vi "单参数加标流程.vi"(10 "流程类型":T4, 11 "Slave ID":T6=enum."氨氮") -> ()   [LabVIEW 2016, in "质控单元V4.lvlib"]
panel:
  in  "平行样测试数据":T1={"时间"=timestamp(0 s since 1904-01-01), "参数"="", "数据类型"="N", "第一次水样浓度值"=0.0, "第二次水样测试时间"=timestamp(0 s since 1904-01-01), "第二次水样浓度值"=0.0}
  in  "集成干预测试数据":T2={"时间"=timestamp(0 s since 1904-01-01), "参数"="", "数据类型"="N", "集成干预测试浓度值"=0.0, "集成干预前测试时间"=timestamp(0 s since 1904-01-01), "集成干预前测试浓度值"=0.0}
  out "平行样启动时间":timestamp
  out "加标模块润洗流程控制":T3=enum."启动水样润洗流程"
  in  "获取加标回收测试数据计数":u16
  in  "获取水样测试数据计数":u16
  in  "写入加标体积重试次数":u16
  in  "加标模块加标润洗启动计数":u16
  out "加标回收启动时间":timestamp
  out "水样测试启动时间":timestamp
  out "Next State":string
  in  "仪器加标回收启动计数":u16
  in  "仪器水样测试启动计数":u16
  in  "加标模块排液启动计数":u16
  in  "加标模块加标启动计数":u16
  in  "加标模块进样启动计数":u16
  in  "加标模块水样润洗启动计数":u16
  in  "采配水启动次数计数":u16
  in  "加标回收测试时间":timestamp
  in  "水样测试时间":timestamp
  in  "质控数据":T5
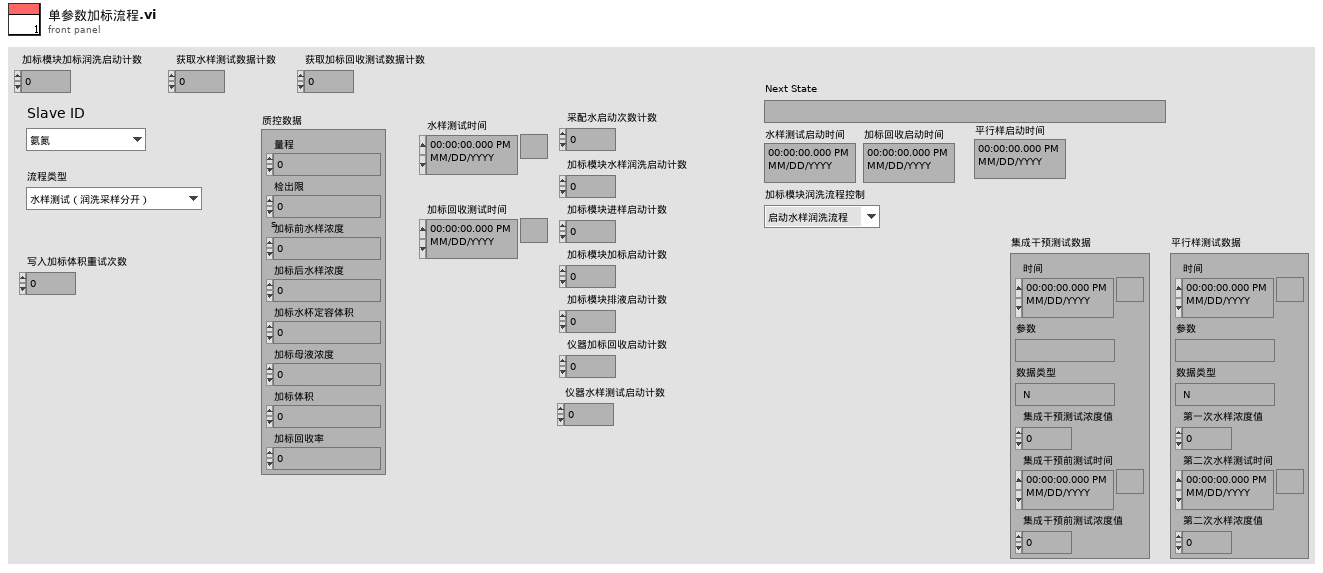
[diagram p1: front panel]
types:
  T1 = typedef "平行样测试数据字段定义.ctl" = cluster{"时间":timestamp, "参数":string, "数据类型":string, "第一次水样浓度值":dbl, "第二次水样测试时间":timestamp, "第二次水样浓度值":dbl}
  T2 = typedef "集成干预字段定义.ctl" = cluster{"时间":timestamp, "参数":string, "数据类型":string, "集成干预测试浓度值":dbl, "集成干预前测试时间":timestamp, "集成干预前测试浓度值":dbl}
  T3 = typedef "质控单元V4.lvlib/质控流程控制.ctl" = enum16{"待机", "启动进样流程", "启动加标流程", "启动排液流程", "启动水样润洗流程", "启动加标润洗流程", "停止流程"}
  T4 = typedef "质控单元V4.lvlib/测试子流程.ctl" = enum16{"水样测试（润洗采样分开）", "水样测试（润洗采样合并）", "水样测试（不启动采配水）", "加标回收（润洗采样分开）", "加标回收（润洗采样合并）", "加标回收（不启动采配水）", "集成干预测试", "平行样测试", "平行样测试（不启动采配水）", "水样测试（不含采样杯）", "平行样测试（不含采样杯）", "集成干预测试（不含采样杯）"}
  T5 = cluster{"量程":dbl, "检出限":dbl, "加标前水样浓度":dbl, "加标后水样浓度":dbl, "加标水杯定容体积":dbl, "加标母液浓度":dbl, "加标体积":dbl, "加标回收率":dbl}
  T6 = typedef "质控单元V4.lvlib/质控slave id.ctl" = enum16{"null", "氨氮", "总磷", "总氮", "CODMn", "CODCr"}
  T7 = cluster{"氨氮":bool, "总磷":bool, "总氮":bool, "CODMn":bool, "CODCr":bool}
  T8 = cluster{"时间":timestamp, "参数":string, "数据类型":string, "加标回收率":sgl, "加标前水样测试时间":timestamp, "加标前水样浓度值":sgl, "加标后水样浓度值":sgl, "加标母液浓度值":sgl, "加标体积":sgl, "加标水杯定容体积":sgl}
  T9 = enum16{"待机", "水样测试（全流程）", "停止", "加标回收", "水样测试（简易流程）"}
  T10 = enum16{"待机", "润洗", "采样", "沉淀", "配水", "反冲洗", "储水", "结束"}
  T11 = typedef "质控单元V4.lvlib/采配水通用流程.ctl" = enum16{"待机", "润洗", "采样", "沉淀", "配水", "反冲洗", "结束"}
  T12 = typedef "质控单元V4.lvlib/质控组合命令区.ctl" = enum16{"停止", "进水样", "排废液", "进空气（搅拌）", "定量（反转定量）"}
  T13 = enum16{"待机", "润洗", "进样", "定量", "加标", "等待取样", "排液", "异常停机"}
  T14 = enum16{"空闲", "水样测试", "标样核查", "零点核查", "跨度核查", "空白测试", "平行样测试", "加标回收", "空白校准", "标样校准", "初始化（清洗）"}
  T15 = cluster{"水样数据时间":timestamp, "水样实测值":sgl, "水样数据标识":string}
  T16 = cluster{"时间":timestamp, "参数":string, "数据类型":string, "第一次水样浓度值":dbl, "第二次水样测试时间":timestamp, "第二次水样浓度值":dbl}
  T17 = typedef "数据库类型.ctl" = enum16{"Access", "SQLite"}
  T18 = cluster{"加标回收数据时间":timestamp, "加标回收实测值":sgl, "加标回收数据标识":string}
  T19 = typedef "质控单元V4.lvlib/质控仪器状态.ctl" = cluster{"运行状态":enum16{"待机", "润洗", "进样", "定量", "加标", "等待取样", "排液", "异常停机"}, "液位状态":enum16{"无感应", "有感应"}, "告警状态":enum16{"无告警", "液位故障告警", "注射泵异常"}, "当前步骤数":u16, "当前步骤剩余时间":u16, "当前步骤具体操作":enum16{"加标", "进样", "排液", "搅拌", "定量"}, "当前流程":enum16{"待机", "进样流程", "加标流程", "排液流程", "水样润洗流程", "加标润洗流程"}}
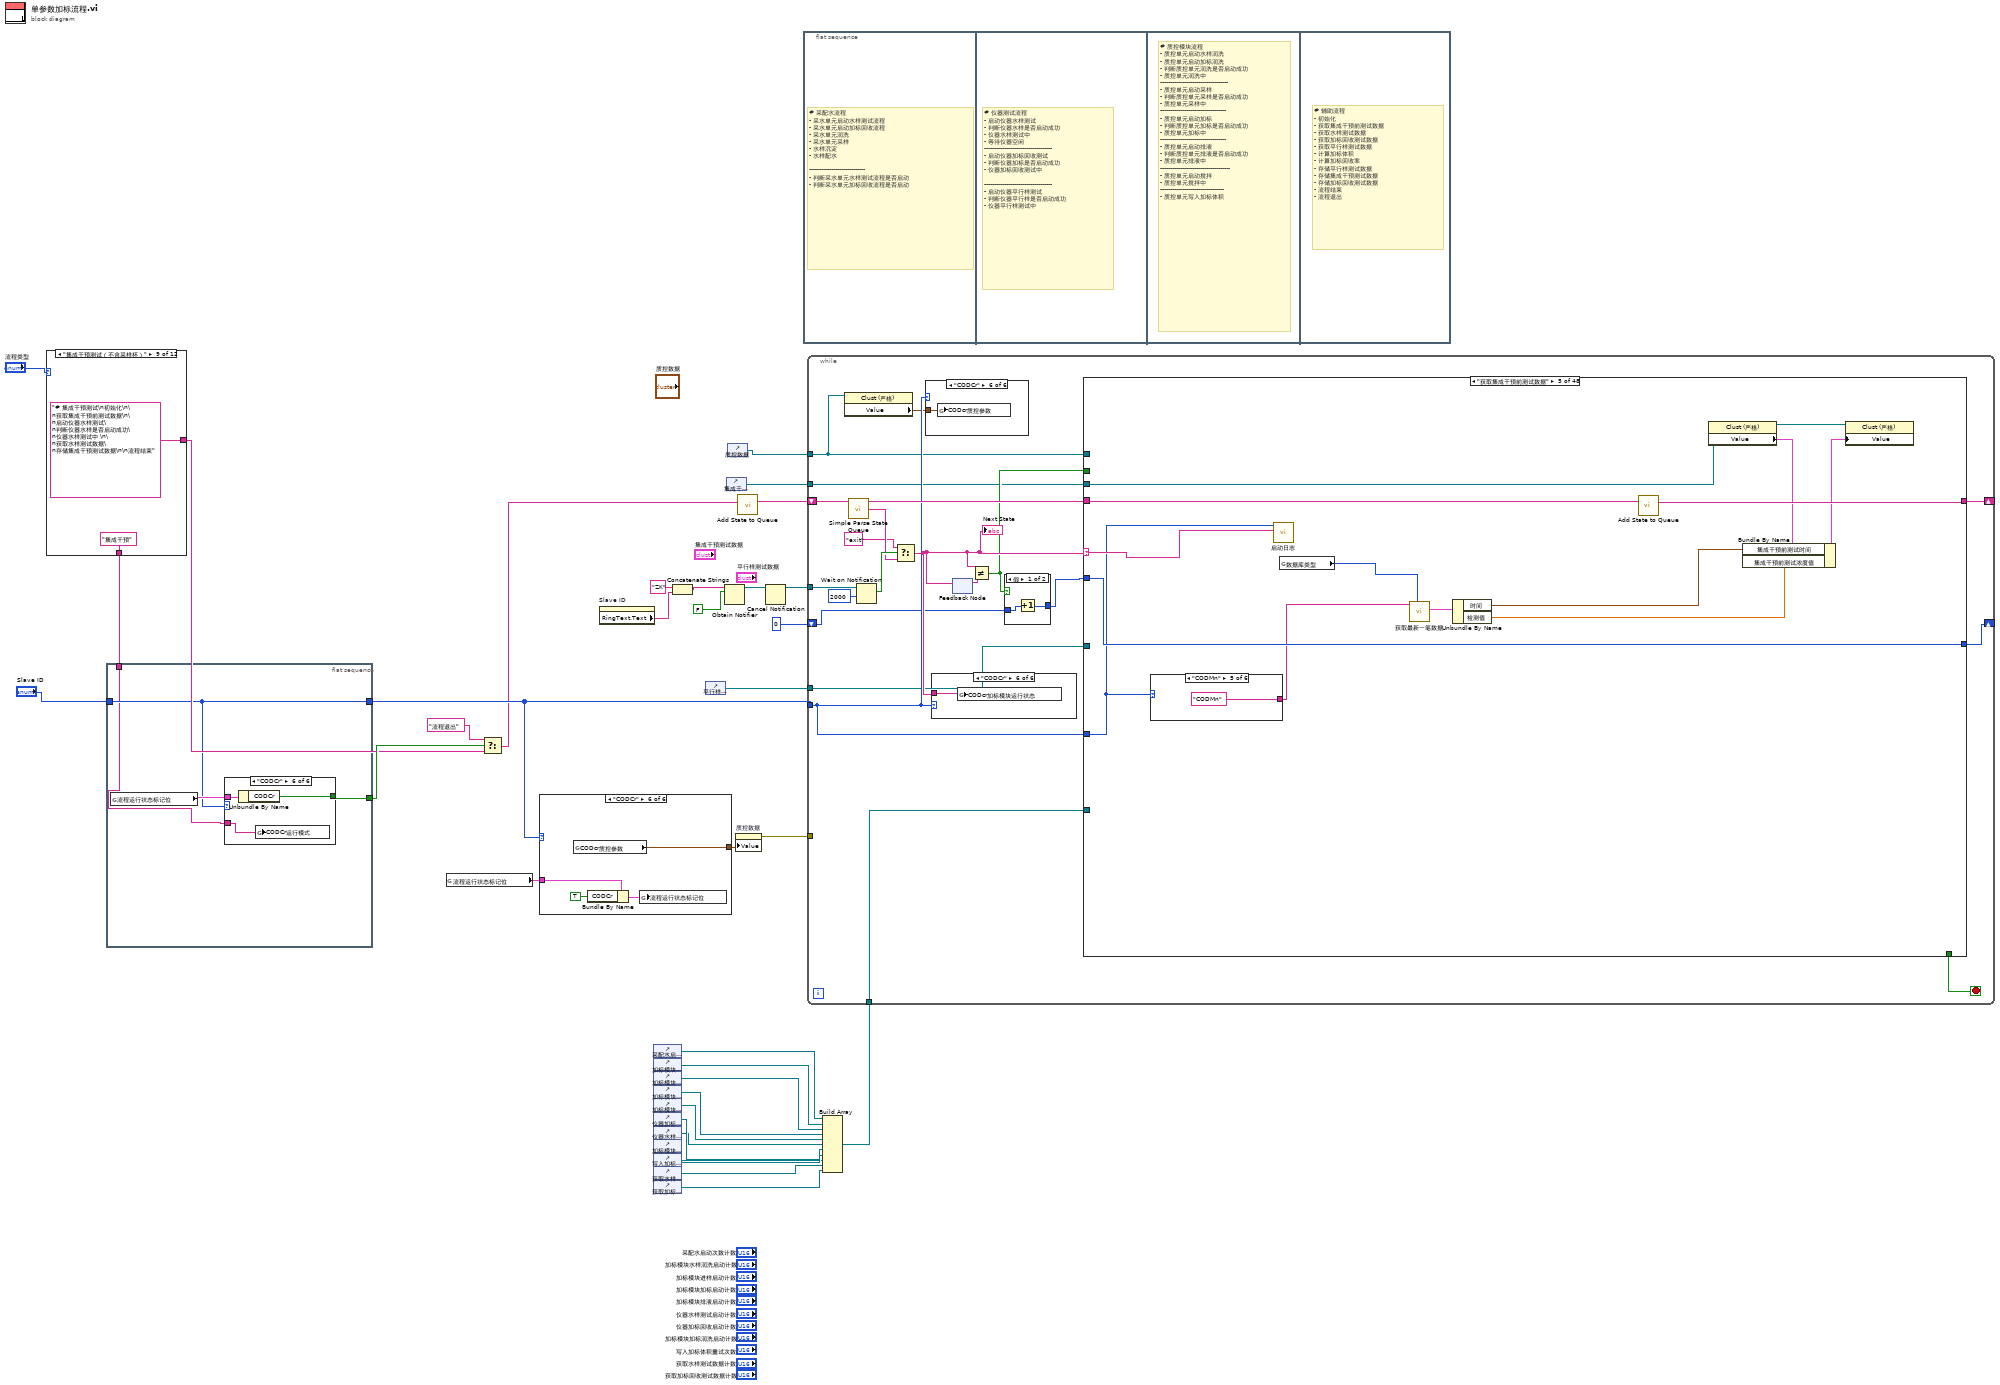
[diagram p0: block diagram]
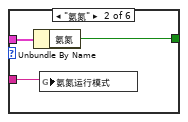
[diagram p3: hidden frame]
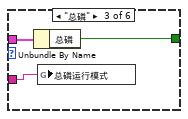
[diagram p4: hidden frame]
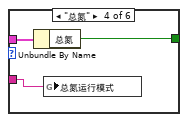
[diagram p5: hidden frame]
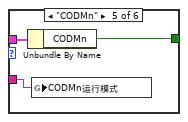
[diagram p6: hidden frame]
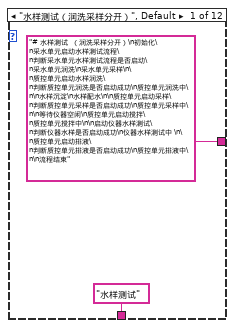
[diagram p7: hidden frame]
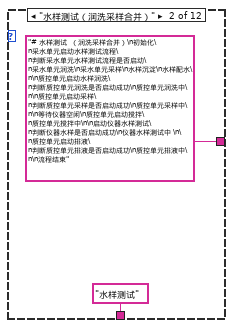
[diagram p8: hidden frame]
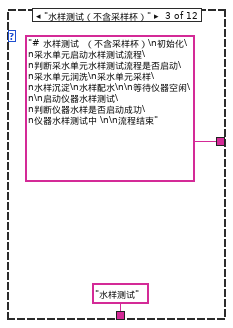
[diagram p9: hidden frame]
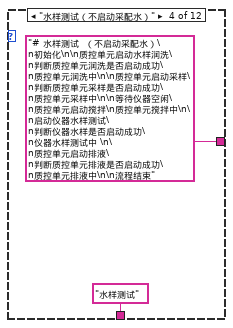
[diagram p10: hidden frame]
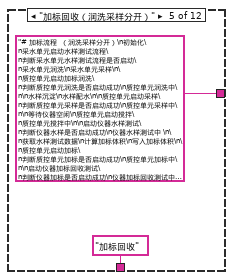
[diagram p11: hidden frame]
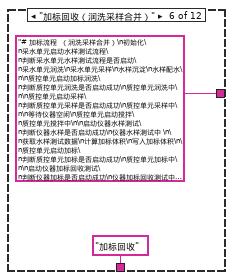
[diagram p12: hidden frame]
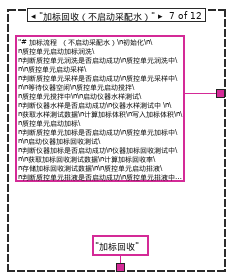
[diagram p13: hidden frame]
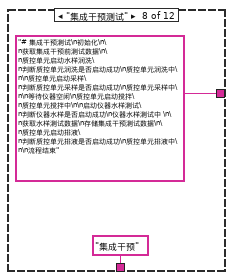
[diagram p14: hidden frame]
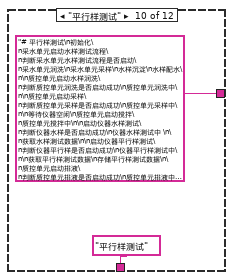
[diagram p15: hidden frame]
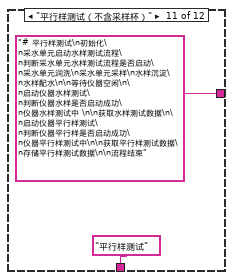
[diagram p16: hidden frame]
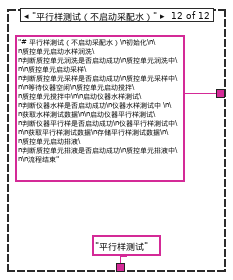
[diagram p17: hidden frame]
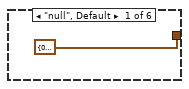
[diagram p18: hidden frame]
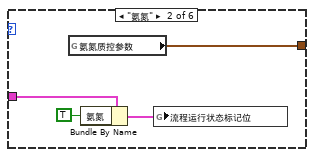
[diagram p19: hidden frame]
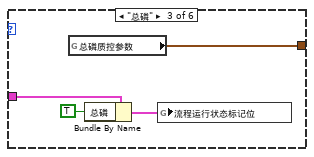
[diagram p20: hidden frame]
diagram:
  n1 = case shown="\"集成干预测试（不含采样杯）\"" "流程类型" {
    tunnel: ["# 水样测试  （润洗采样分开）\n初始化\n采水单元启动水样测试流程\n判断采水单元水样测试流程是否启动\n采水单元润洗\n采水单元采样\n\n质控单元启动水样润洗\n判断质控单元润洗是否启动成功\n质控单元润洗中\n\n水样沉淀\n水样配水\n\n质控单元启动采样\n判断质控单元采样是否启动成功\n质控单元采样中\n\n等待仪器空闲\n质控单元启动搅拌\n质控单元搅拌中\n\n启动仪器水样测试\n判断仪器水样是否启动成功\n仪器水样测试中 \n\n质控单元启动排液\n判断质控单元排液是否启动成功\n质控单元排液中\n\n流程结束" ("State(s) In (\"\")") "# 水样测试  （润洗采样合并）\n初始化\n采水单元启动水样测试流程\n判断采水单元水样测试流程是否启动\n采水单元润洗\n采水单元采样\n水样沉淀\n水样配水\n\n质控单元启动水样润洗\n判断质控单元润洗是否启动成功\n质控单元润洗中\n\n质控单元启动采样\n判断质控单元采样是否启动成功\n质控单元采样中\n\n等待仪器空闲\n质控单元启动搅拌\n质控单元搅拌中\n\n启动仪器水样测试\n判断仪器水样是否启动成功\n仪器水样测试中 \n\n质控单元启动排液\n判断质控单元排液是否启动成功\n质控单元排液中\n\n流程结束" ("State(s) In (\"\")") "# 水样测试  （不含采样杯）\n初始化\n采水单元启动水样测试流程\n判断采水单元水样测试流程是否启动\n采水单元润洗\n采水单元采样\n水样沉淀\n水样配水\n\n等待仪器空闲\n\n启动仪器水样测试\n判断仪器水样是否启动成功\n仪器水样测试中 \n\n流程结束" ("State(s) In (\"\")") "# 水样测试  （不启动采配水）\n初始化\n\n质控单元启动水样润洗\n判断质控单元润洗是否启动成功\n质控单元润洗中\n\n质控单元启动采样\n判断质控单元采样是否启动成功\n质控单元采样中\n\n等待仪器空闲\n质控单元启动搅拌\n质控单元搅拌中\n\n启动仪器水样测试\n判断仪器水样是否启动成功\n仪器水样测试中 \n\n质控单元启动排液\n判断质控单元排液是否启动成功\n质控单元排液中\n\n流程结束" ("State(s) In (\"\")") "# 加标流程  （润洗采样分开）\n初始化\n采水单元启动水样测试流程\n判断采水单元水样测试流程是否启动\n采水单元润洗\n采水单元采样\n\n质控单元启动加标润洗\n判断质控单元润洗是否启动成功\n质控单元润洗中\n\n水样沉淀\n水样配水\n\n质控单元启动采样\n判断质控单元采样是否启动成功\n质控单元采样中\n\n等待仪器空闲\n质控单元启动搅拌\n质控单元搅拌中\n\n启动仪器水样测试\n判断仪器水样是否启动成功\n仪器水样测试中 \n\n获取水样测试数据\n计算加标体积\n写入加标体积\n\n质控单元启动加标\n判断质控单元加标是否启动成功\n质控单元加标中\n\n启动仪器加标回收测试\n判断仪器加标是否启动成功\n仪器加标回收测试中\n\n获取加标回收测试数据\n计算加标回收率\n存储加标回收测试数据\n\n质控单元启动排液\n判断质控单元排液是否启动成功\n质控单元排液中\n\n流程结束" ("State(s) In (\"\")") "# 加标流程  （润洗采样合并）\n初始化\n采水单元启动水样测试流程\n判断采水单元水样测试流程是否启动\n采水单元润洗\n采水单元采样\n水样沉淀\n水样配水\n\n质控单元启动加标润洗\n判断质控单元润洗是否启动成功\n质控单元润洗中\n\n质控单元启动采样\n判断质控单元采样是否启动成功\n质控单元采样中\n\n等待仪器空闲\n质控单元启动搅拌\n质控单元搅拌中\n\n启动仪器水样测试\n判断仪器水样是否启动成功\n仪器水样测试中 \n\n获取水样测试数据\n计算加标体积\n写入加标体积\n\n质控单元启动加标\n判断质控单元加标是否启动成功\n质控单元加标中\n\n启动仪器加标回收测试\n判断仪器加标是否启动成功\n仪器加标回收测试中\n\n获取加标回收测试数据\n计算加标回收率\n存储加标回收测试数据\n\n质控单元启动排液\n判断质控单元排液是否启动成功\n质控单元排液中\n\n流程结束" ("State(s) In (\"\")") "# 加标流程  （不启动采配水）\n初始化\n\n质控单元启动加标润洗\n判断质控单元润洗是否启动成功\n质控单元润洗中\n\n质控单元启动采样\n判断质控单元采样是否启动成功\n质控单元采样中\n\n等待仪器空闲\n质控单元启动搅拌\n质控单元搅拌中\n\n启动仪器水样测试\n判断仪器水样是否启动成功\n仪器水样测试中 \n\n获取水样测试数据\n计算加标体积\n写入加标体积\n\n质控单元启动加标\n判断质控单元加标是否启动成功\n质控单元加标中\n\n启动仪器加标回收测试\n判断仪器加标是否启动成功\n仪器加标回收测试中\n\n获取加标回收测试数据\n计算加标回收率\n存储加标回收测试数据\n\n质控单元启动排液\n判断质控单元排液是否启动成功\n质控单元排液中\n\n流程结束" ("State(s) In (\"\")") "# 集成干预测试\n初始化\n\n获取集成干预前测试数据\n\n质控单元启动水样润洗\n判断质控单元润洗是否启动成功\n质控单元润洗中\n\n质控单元启动采样\n判断质控单元采样是否启动成功\n质控单元采样中\n\n等待仪器空闲\n质控单元启动搅拌\n质控单元搅拌中\n\n启动仪器水样测试\n判断仪器水样是否启动成功\n仪器水样测试中 \n\n获取水样测试数据\n存储集成干预测试数据\n\n质控单元启动排液\n判断质控单元排液是否启动成功\n质控单元排液中\n\n流程结束" ("State(s) In (\"\")") "# 集成干预测试\n初始化\n\n获取集成干预前测试数据\n\n启动仪器水样测试\n判断仪器水样是否启动成功\n仪器水样测试中 \n\n获取水样测试数据\n存储集成干预测试数据\n\n流程结束" ("State(s) In (\"\")") "# 平行样测试\n初始化\n采水单元启动水样测试流程\n判断采水单元水样测试流程是否启动\n采水单元润洗\n采水单元采样\n水样沉淀\n水样配水\n\n质控单元启动水样润洗\n判断质控单元润洗是否启动成功\n质控单元润洗中\n\n质控单元启动采样\n判断质控单元采样是否启动成功\n质控单元采样中\n\n等待仪器空闲\n质控单元启动搅拌\n质控单元搅拌中\n\n启动仪器水样测试\n判断仪器水样是否启动成功\n仪器水样测试中 \n\n获取水样测试数据\n\n启动仪器平行样测试\n判断仪器平行样是否启动成功\n仪器平行样测试中\n\n获取平行样测试数据\n存储平行样测试数据\n\n质控单元启动排液\n判断质控单元排液是否启动成功\n质控单元排液中\n\n流程结束" ("State(s) In (\"\")") "# 平行样测试\n初始化\n采水单元启动水样测试流程\n判断采水单元水样测试流程是否启动\n采水单元润洗\n采水单元采样\n水样沉淀\n水样配水\n\n等待仪器空闲\n\n启动仪器水样测试\n判断仪器水样是否启动成功\n仪器水样测试中 \n\n获取水样测试数据\n\n启动仪器平行样测试\n判断仪器平行样是否启动成功\n仪器平行样测试中\n\n获取平行样测试数据\n存储平行样测试数据\n\n流程结束" ("State(s) In (\"\")") "# 平行样测试（不启动采配水）\n初始化\n\n质控单元启动水样润洗\n判断质控单元润洗是否启动成功\n质控单元润洗中\n\n质控单元启动采样\n判断质控单元采样是否启动成功\n质控单元采样中\n\n等待仪器空闲\n质控单元启动搅拌\n质控单元搅拌中\n\n启动仪器水样测试\n判断仪器水样是否启动成功\n仪器水样测试中 \n\n获取水样测试数据\n\n启动仪器平行样测试\n判断仪器平行样是否启动成功\n仪器平行样测试中\n\n获取平行样测试数据\n存储平行样测试数据\n\n质控单元启动排液\n判断质控单元排液是否启动成功\n质控单元排液中\n\n流程结束" ("State(s) In (\"\")")] -> w12
    tunnel: ["水样测试" "水样测试" "水样测试" "水样测试" "加标回收" "加标回收" "加标回收" "集成干预" "集成干预" "平行样测试" "平行样测试" "平行样测试"] -> w6
    frame "水样测试（润洗采样分开）", Default {
    }
    frame "水样测试（润洗采样合并）" {
    }
    frame "水样测试（不含采样杯）" {
    }
    frame "水样测试（不启动采配水）" {
    }
    frame "加标回收（润洗采样分开）" {
    }
    frame "加标回收（润洗采样合并）" {
    }
    frame "加标回收（不启动采配水）" {
    }
    frame "集成干预测试" {
    }
    frame "集成干预测试（不含采样杯）" {
    }
    frame "平行样测试" {
    }
    frame "平行样测试（不含采样杯）" {
    }
    frame "平行样测试（不启动采配水）" {
    }
  }
  n2 = flat-sequence {
    tunnel: [w60] -> w15
    tunnel: [w61] -> w14
    tunnel: "Slave ID" -> [w60]
    tunnel: w6 -> [w59]
    frame #0 {
      n3 = global read "ZK非断电保存全局变量.vi" "流程运行状态标记位"() -> (w62:T7)
      n4 = case shown="\"CODCr\"" w60 {
        tunnel: w62 -> [_ w65 w68 w71 w74 w77]
        tunnel: [_ w64 w67 w70 w73 w76] -> w61
        tunnel: w59 -> [_ w63 w66 w69 w72 w75]
        frame "null", Default {
        }
        frame "氨氮" {
          n5 = Unbundle By Name(w65) -> ("氨氮"=w64:bool)
          n6 = global write "ZK非断电保存全局变量.vi" "氨氮运行模式"(w63) -> ()
        }
        frame "总磷" {
          n7 = Unbundle By Name(w68) -> ("总磷"=w67:bool)
          n8 = global write "ZK非断电保存全局变量.vi" "总磷运行模式"(w66) -> ()
        }
        frame "总氮" {
          n9 = Unbundle By Name(w71) -> ("总氮"=w70:bool)
          n10 = global write "ZK非断电保存全局变量.vi" "总氮运行模式"(w69) -> ()
        }
        frame "CODMn" {
          n11 = Unbundle By Name(w74) -> ("CODMn"=w73:bool)
          n12 = global write "ZK非断电保存全局变量.vi" "CODMn运行模式"(w72) -> ()
        }
        frame "CODCr" {
          n13 = Unbundle By Name(w77) -> ("CODCr"=w76:bool)
          n14 = global write "ZK非断电保存全局变量.vi" "CODCr运行模式"(w75) -> ()
        }
      }
    }
  }
  n15 = global read "ZK非断电保存全局变量.vi" "流程运行状态标记位"() -> (w17:T7)
  n16 = Select(t="流程退出", s=w14, f=w12) -> (s? t:f=w11:string)
  n17 = case shown="\"CODCr\"" w15 {
    tunnel: [T5 {"量程"=0.0, "检出限"=0.0, "加标前水样浓度"=0.0, "加标后水样浓度"=0.0, "加标水杯定容体积"=0.0, "加标母液浓度"=0.0, "加标体积"=0.0, "加标回收率"=0.0} ("CODcr质控参数") w82 w86 w90 w94 w98] -> w26
    tunnel: w17 -> [_ w81 w83 w87 w91 w95]
    frame "null", Default {
    }
    frame "氨氮" {
      n18 = global read "ZK断电保存全局变量.vi" "氨氮质控参数"() -> (w82:T5)
      n19 = Bundle By Name(cluster=w81, "氨氮"=TRUE) -> (w80:T7)
      n20 = global write "ZK非断电保存全局变量.vi" "流程运行状态标记位"(w80) -> ()
    }
    frame "总磷" {
      n21 = global read "ZK断电保存全局变量.vi" "总磷质控参数"() -> (w86:T5)
      n22 = Bundle By Name(cluster=w83, "总磷"=TRUE ("氨氮")) -> (w85:T7)
      n23 = global write "ZK非断电保存全局变量.vi" "流程运行状态标记位"(w85) -> ()
    }
    frame "总氮" {
      n24 = global read "ZK断电保存全局变量.vi" "总氮质控参数"() -> (w90:T5)
      n25 = Bundle By Name(cluster=w87, "总氮"=TRUE ("氨氮")) -> (w89:T7)
      n26 = global write "ZK非断电保存全局变量.vi" "流程运行状态标记位"(w89) -> ()
    }
    frame "CODMn" {
      n27 = global read "ZK断电保存全局变量.vi" "CODMn质控参数"() -> (w94:T5)
      n28 = Bundle By Name(cluster=w91, "CODMn"=TRUE ("氨氮")) -> (w93:T7)
      n29 = global write "ZK非断电保存全局变量.vi" "流程运行状态标记位"(w93) -> ()
    }
    frame "CODCr" {
      n30 = global read "ZK断电保存全局变量.vi" "CODcr质控参数"() -> (w98:T5)
      n31 = Bundle By Name(cluster=w95, "CODCr"=TRUE ("氨氮")) -> (w97:T7)
      n32 = global write "ZK非断电保存全局变量.vi" "流程运行状态标记位"(w97) -> ()
    }
  }
  n33 = property on="Slave ID" class="Enum (严格)"() -> ("RingText.Text"=w34:string)  [unwired: 2 in, 2 out]
  n34 = control-ref of="采配水启动次数计数"() -> (w24:refnum<vi>)
  n35 = control-ref of="加标模块水样润洗启动计数"() -> (w23:refnum<vi>)
  n36 = control-ref of="加标模块进样启动计数"() -> (w22:refnum<vi>)
  n37 = control-ref of="加标模块加标启动计数"() -> (w21:refnum<vi>)
  n38 = control-ref of="加标模块排液启动计数"() -> (w20:refnum<vi>)
  n39 = control-ref of="仪器加标回收启动计数"() -> (w5:refnum<vi>)
  n40 = control-ref of="仪器水样测试启动计数"() -> (w4:refnum<vi>)
  n41 = control-ref of="加标模块加标润洗启动计数"() -> (w16:refnum<vi>)
  n42 = control-ref of="写入加标体积重试次数"() -> (w10:refnum<vi>)
  n43 = control-ref of="获取水样测试数据计数"() -> (w9:refnum<vi>)
  n44 = control-ref of="获取加标回收测试数据计数"() -> (w8:refnum<vi>)
  n45 = Concatenate Strings("ZK" ("字符串"), w34) -> (w32:string)
  n46 = control-ref of="平行样测试数据"() -> (w1:refnum<vi>)
  n47 = Obtain Notifier(name (unnamed)=w32, notification data type=FALSE) -> (notifier out=w30:refnum<notifier>)  [unwired: 2 in, 2 out]
  n48 = control-ref of="集成干预测试数据"() -> (w2:refnum<vi>)
  n49 = control-ref of="质控数据"() -> (w25:refnum<vi>)
  n50 = property on="质控数据" class="Clust (严格)"("Value"=w26) -> (error out=w27:errorcluster)  [unwired: 2 in, 1 out]
  n51 = call "Add State to Queue.vi"("State(s) In (\"\")"=w11) -> ("States Out"=w28:string)  [unwired: 14 in]
  n52 = Cancel Notification(0:w30) -> (8:w29:refnum<notifier>)  [unwired: 1 in, 2 out]
  n53 = flat-sequence {
    frame #0 {
      # "# 采配水流程\n- 采水单元启动水样测试流程\n- 采水单元启动加标回收流程\n- 采水单元润洗\n- 采水单元采样 \n- 水样沉淀\n- 水样配水\n\n----------------------------\n- 判断采水单元水样测试流程是否启动\n- 判断采水单元加标回收流程是否启动"
    }
    frame #1 {
      # "# 仪器测试流程\n- 启动仪器水样测试\n- 判断仪器水样是否启动成功\n- 仪器水样测试中\n- 等待仪器空闲\n----------------------------------\n- 启动仪器加标回收测试\n- 判断仪器加标是否启动成功\n- 仪器加标回收测试中\n\n----------------------------------\n- 启动仪器平行样测试\n- 判断仪器平行样是否启动成功\n- 仪器平行样测试中"
    }
    frame #2 {
      # "# 质控模块流程\n- 质控单元启动水样润洗\n- 质控单元启动加标润洗\n- 判断质控单元润洗是否启动成功\n- 质控单元润洗中\n----------------------------------\n- 质控单元启动采样\n- 判断质控单元采样是否启动成功\n- 质控单元采样中\n---------------------------------\n- 质控单元启动加标\n- 判断质控单元加标是否启动成功\n- 质控单元加标中\n---------------------------------\n- 质控单元启动排液\n- 判断质控单元排液是否启动成功\n- 质控单元排液中\n-----------------------------------\n- 质控单元启动搅拌\n- 质控单元搅拌中\n--------------------------------\n- 质控单元写入加标体积"
    }
    frame #3 {
      # "# 辅助流程\n- 初始化\n- 获取集成干预前测试数据\n- 获取水样测试数据\n- 获取加标回收测试数据\n- 获取平行样测试数据\n- 计算加标体积\n- 计算加标回收率\n- 存储平行样测试数据\n- 存储集成干预测试数据\n- 存储加标回收测试数据 \n- 流程结束\n- 流程退出"
    }
  }
  n54 = Build Array(w24, w23, w22, w21, w20, w4, w5, w16, w10, w9, w8) -> (w19:refnum<vi>[])
  n55 = while {
    tunnel: w29 -> [w118]
    tunnel: w15 -> [w110]
    shift-right: [w112] -> _
    shift-left: w28 -> [w119]
    tunnel: w27 -> [_]
    tunnel: w25 -> [w109]
    tunnel: w19 -> [w107]
    shift-right: [w102] -> _
    shift-left: 0 -> [w104]
    tunnel: w2 -> [w99]
    tunnel: w1 -> [w100]
    stop <- w111 stop-if-true
    n56 = property class="Clust (严格)"(reference=w109) -> ("Value"=w108:T5)  [unwired: 1 in, 2 out]
    n57 = call "Simple Parse State Queue.vi"("State Queue"=w119) -> ("Remain States"=w113:string, "Next State"=w115:string)  [unwired: 13 in]
    n58 = Wait on Notification(notifier=w118, timeout in ms (-1)=2000 ("超时毫秒(-1)")) -> (notification=w116:bool)  [unwired: 2 in, 3 out]
    n59 = Select(t="exit" ("State(s) In (\"\")"), s=w116, f=w115) -> (s? t:f=w105:string)
    "Next State" <- w105
    n60 = case shown="\"CODCr\"" w110 {
      tunnel: w108 -> [_ w122 w123 w124 w125 w126]
      frame "null", Default {
      }
      frame "氨氮" {
        n61 = global write "ZK断电保存全局变量.vi" "氨氮质控参数"(w122) -> ()
      }
      frame "总磷" {
        n62 = global write "ZK断电保存全局变量.vi" "总磷质控参数"(w123) -> ()
      }
      frame "总氮" {
        n63 = global write "ZK断电保存全局变量.vi" "总氮质控参数"(w124) -> ()
      }
      frame "CODMn" {
        n64 = global write "ZK断电保存全局变量.vi" "CODMn质控参数"(w125) -> ()
      }
      frame "CODCr" {
        n65 = global write "ZK断电保存全局变量.vi" "CODcr质控参数"(w126) -> ()
      }
    }
    n66 = case shown="\"CODCr\"" w110 {
      tunnel: w105 -> [_ w127 w128 w129 w130 w131]
      frame "null", Default {
      }
      frame "氨氮" {
        n67 = global write "ZK非断电保存全局变量.vi" "氨氮加标模块运行状态"(w127) -> ()
      }
      frame "总磷" {
        n68 = global write "ZK非断电保存全局变量.vi" "总磷加标模块运行状态"(w128) -> ()
      }
      frame "总氮" {
        n69 = global write "ZK非断电保存全局变量.vi" "总氮加标模块运行状态"(w129) -> ()
      }
      frame "CODMn" {
        n70 = global write "ZK非断电保存全局变量.vi" "CODMn加标模块运行状态"(w130) -> ()
      }
      frame "CODCr" {
        n71 = global write "ZK非断电保存全局变量.vi" "CODcr加标模块运行状态"(w131) -> ()
      }
    }
    n72 = feedback-in #1(w105) -> ()
    n73 = feedback #1() -> (w106:string)  [unwired: 1 in]
    n74 = Not Equal?(x=w105, y=w106) -> (x != y?=w101:bool)
    n75 = case shown="假" w101 {
      tunnel: w104 -> [w121 _]
      tunnel: [w120 _] -> w103
      frame False {
        n76 = Increment(x=w121) -> (x+1=w120:i32)
      }
      frame True {
      }
    }
    n77 = case shown="\"获取集成干预前测试数据\"" w105 {
      selector: w105 -> [_ _ w143 w168 w226 w236 w290 w341 w351 w362 w389 w406 w418 w448 _ w458 w469 w481 w502 w524 w545 w566 w588 _ w605 w618 w629 w647 w667 w679 w694 w702 w735 w767 w799 w836 w865 w897 _ w912 w929 w947 w965 w984 w1017 w1049 w1081 w1114]
      tunnel: w113 -> [w134 w137 w152 w190 w228 w262 w314 w349 w358 w376 w392 w408 w424 w452 w455 w466 w477 w496 w503 w536 w554 w574 w596 w603 w615 w627 w639 w654 w677 w689 w696 w716 w750 w782 w814 w845 w875 w900 w908 w921 w933 w956 w974 w986 w1032 w1064 w1096 w1120]
      tunnel: [w133 w136 w151 w189 w227 w261 w313 w348 w357 w375 w391 w407 w423 w451 w454 w465 w476 w495 w517 w535 w553 w573 w595 w602 w614 w626 w638 w653 w676 w688 w695 w715 w749 w781 w813 w844 w874 w899 w907 w920 w932 w955 w973 w985 w1031 w1063 w1095 w1119] -> w112
      tunnel: [_ _ _ _ _ _ _ _ _ _ _ _ TRUE TRUE _ _ _ _ _ _ _ _ _ _ _ _ _ _ _ _ _ _ _ _ _ _ _ _ _ _ _ _ _ _ _ _ _ _] -> w111
      tunnel: w110 -> [_ _ w142 w177 w220 w247 w301 w340 w352 w363 w390 w401 w419 w449 _ w459 w470 w480 w501 w523 w543 w563 w586 _ w606 w619 w630 w641 w668 w680 w691 w700 w733 w765 w797 w830 w863 w892 _ w913 w930 w948 w966 w982 w1015 w1047 w1079 w1113]
      tunnel: w109 -> [_ _ w148 w188 _ w260 _ w347 w356 w374 _ _ _ _ _ _ _ _ _ _ _ _ _ _ _ _ _ w652 _ _ _ _ _ _ _ _ _ _ _ _ _ _ _ _ _ _ _ _]
      tunnel: w107 -> [_ _ w139 w174 _ w238 w292 _ _ _ _ _ _ _ _ w464 w475 w485 w507 _ _ _ _ _ w608 w621 w632 w646 w671 w683 _ w706 w739 w771 w803 _ _ _ _ w916 _ w951 w969 _ w1021 w1054 w1086 _]
      tunnel: w103 -> [w132 w135 w138 w165 w225 w235 w289 w339 w350 w359 w388 w405 w415 w445 w453 w457 w468 w478 w499 w521 w542 w561 w585 w601 w604 w616 w628 w640 w666 w678 w690 w697 w732 w764 w796 w829 w862 w895 w906 w910 w931 w945 w963 w981 w1014 w1046 w1078 w1111]
      tunnel: [w132 w135 w138 w165 w225 w235 w289 w339 w350 w359 w388 w405 w415 w445 w453 w457 w468 w478 w499 w521 w542 w561 w585 w601 w604 w616 w628 w640 w666 w678 w690 w697 w732 w764 w796 w829 w862 w895 w906 w910 w931 w945 w963 w981 w1014 w1046 w1078 w1111] -> w102
      tunnel: w101 -> [_ _ _ _ _ _ _ _ _ _ _ _ _ _ _ _ _ _ _ w520 w541 w560 w584 _ _ _ _ _ _ _ _ _ _ _ _ w828 w861 w891 _ _ w927 _ _ _ _ _ _ w1110]
      tunnel: w100 -> [_ _ _ w163 _ _ w288 _ _ _ w387 _ _ _ _ _ _ _ _ _ _ _ _ _ _ _ _ _ _ _ _ _ _ _ _ _ _ _ _ _ _ _ _ _ _ _ _ _]
      tunnel: w99 -> [_ _ _ w157 w221 _ _ _ _ _ _ w404 _ _ _ _ _ _ _ _ _ _ _ _ _ _ _ _ _ _ _ _ _ _ _ _ _ _ _ _ _ _ _ _ _ _ _ _]
      frame Default {
        n78 = call "Add State to Queue.vi"("State(s) In (\"\")"=w134) -> ("States Out"=w133:string)  [unwired: 14 in]
      }
      frame "-------------------# 辅助流程 #-------------------" {
        n79 = call "Add State to Queue.vi"("State(s) In (\"\")"=w137) -> ("States Out"=w136:string)  [unwired: 14 in]
      }
      frame "初始化" {
        w144 = 0.0 ("加标前水样浓度")
        n80 = property class="Clust (严格)"(reference=w148) -> (reference out=w147:refnum<vi>, "Value"=w146:T5)  [unwired: 1 in, 1 out]
        n81 = for {
          tunnel: w139 -> [w154] mode=indexing
          n82 = property class="DigNum (严格)"(reference=w154, "Value"=u16 0 ("值")) -> ()  [unwired: 1 in, 2 out]
        }
        n83 = Bundle By Name(cluster=w146, "加标前水样浓度"=w144, "加标后水样浓度"=w144, "加标体积"=w144, "加标回收率"=w144) -> (w145:T5)
        n84 = property class="Clust (严格)"(reference=w147, "Value"=w145) -> ()  [unwired: 1 in, 2 out]
        n85 = Concatenate Strings("----->>" ("字符串"), w143) -> (w141:string)
        n86 = call "ZK报警清除.vi"("Slave ID"=w142) -> ()  [unwired: 10 in, 1 out]
        n87 = call "启动日志.vi"("日志信息"=w141, "Slave ID"=w142) -> ()  [unwired: 9 in, 1 out]
        n88 = call "Add State to Queue.vi"("State(s) In (\"\")"=w152) -> ("States Out"=w151:string)  [unwired: 14 in]
        n89 = local write "水样测试时间"(timestamp(0 s since 1904-01-01) ("水样测试时间")) -> ()
        n90 = local write "加标回收测试时间"(timestamp(0 s since 1904-01-01) ("加标回收测试时间")) -> ()
      }
      frame "获取水样测试数据" {
        n91 = case shown="\"CODCr\"" w177 {
          tunnel: [sgl 0.0 ("水样实测值") w198 w202 w206 w210 w214] -> w155
          tunnel: [timestamp(0 s since 1904-01-01) ("水样数据时间") w197 w201 w205 w209 w213] -> w156
          frame "null", Default {
          }
          frame "氨氮" {
            w195 = u16 3 items=["总磷"=1, "总氮"=2, "氨氮"=3, "CODMn"=21, "CODcr"=22] ("站号")
            n92 = call-poly "获取测试数据.vi"("站号"=w195) -> ("测量数据区"=w196:T15)  [unwired: 10 in]
            n93 = Unbundle By Name(w196) -> ("水样数据时间"=w197:timestamp, "水样实测值"=w198:sgl)
          }
          frame "总磷" {
            w199 = u16 1 items=["总磷"=1, "总氮"=2, "氨氮"=3, "CODMn"=21, "CODcr"=22] ("站号")
            n94 = call-poly "获取测试数据.vi"("站号"=w199) -> ("测量数据区"=w200:T15)  [unwired: 10 in]
            n95 = Unbundle By Name(w200) -> ("水样数据时间"=w201:timestamp, "水样实测值"=w202:sgl)
          }
          frame "总氮" {
            w203 = u16 2 items=["总磷"=1, "总氮"=2, "氨氮"=3, "CODMn"=21, "CODcr"=22] ("站号")
            n96 = call-poly "获取测试数据.vi"("站号"=w203) -> ("测量数据区"=w204:T15)  [unwired: 10 in]
            n97 = Unbundle By Name(w204) -> ("水样数据时间"=w205:timestamp, "水样实测值"=w206:sgl)
          }
          frame "CODMn" {
            w207 = u16 21 items=["总磷"=1, "总氮"=2, "氨氮"=3, "CODMn"=21, "CODcr"=22] ("站号")
            n98 = call-poly "获取测试数据.vi"("站号"=w207) -> ("测量数据区"=w208:T15)  [unwired: 10 in]
            n99 = Unbundle By Name(w208) -> ("水样数据时间"=w209:timestamp, "水样实测值"=w210:sgl)
          }
          frame "CODCr" {
            w211 = u16 22 items=["总磷"=1, "总氮"=2, "氨氮"=3, "CODMn"=21, "CODcr"=22] ("站号")
            n100 = call-poly "获取测试数据.vi"("站号"=w211) -> ("测量数据区"=w212:T15)  [unwired: 10 in]
            n101 = Unbundle By Name(w212) -> ("水样数据时间"=w213:timestamp, "水样实测值"=w214:sgl)
          }
        }
        n102 = Index Array(array=w174, index=9 ("索引")) -> (element=w175:refnum<vi>)
        n103 = property class="DigNum (严格)"(reference=w175) -> (reference out=w173:refnum<vi>, "Value"=w172:u16)  [unwired: 1 in, 1 out]
        n104 = local read "水样测试启动时间"() -> (w184:timestamp)
        n105 = call "启动日志.vi"("日志信息"=w168, "Slave ID"=w177) -> ()  [unwired: 9 in, 1 out]
        n106 = Increment(x=w172) -> (x+1=w171:u16)
        n107 = Subtract(x=w156, y=w184) -> (x-y=w183:dbl)
        n108 = local write "水样测试时间"(w156) -> ()
        n109 = property class="DigNum (严格)"(reference=w173, "Value"=w171) -> ()  [unwired: 1 in, 2 out]
        n110 = Absolute Value(x=w183) -> (abs(x)=w182:dbl)
        n111 = property class="Clust (严格)"(reference=w188) -> (reference out=w187:refnum<vi>, "Value"=w186:T5)  [unwired: 1 in, 1 out]
        n112 = Less Or Equal?(x=w171, y=u16 5) -> (x <= y?=w169:bool)
        n113 = Less?(x=w182, y=300.0) -> (x < y?=w178:bool)
        n114 = Bundle By Name(cluster=w186, "加标前水样浓度"=w155) -> (w185:T5)
        n115 = property class="Clust (严格)"(reference=w187, "Value"=w185) -> ()  [unwired: 1 in, 2 out]
        n116 = Select(t=w168, s=w169, f="exit") -> (s? t:f=w166:string)
        n117 = Select(t="", s=w178, f=w166) -> (s? t:f=w179:string)
        n118 = case shown="假" w178 {
          tunnel: w177 -> [w192 _]
          frame False {
            w191 = "获取水样数据异常" ("日志信息")
            n119 = call "启动日志.vi"("日志信息"=w191, "Slave ID"=w192) -> ()  [unwired: 9 in, 1 out]
            n120 = call "报警信息记录.vi"("报警信息"=w191, "Slave ID"=w192) -> ()  [unwired: 9 in, 1 out]
          }
          frame True {
          }
        }
        n121 = call "Add State to Queue.vi"("State(s) In Front (\"\")"=w179, "State(s) In (\"\")"=w190) -> ("States Out"=w189:string)  [unwired: 13 in]
        n122 = property class="Clust (严格)"(reference=w163) -> (reference out=w164:refnum<vi>, "Value"=w162:T16)  [unwired: 1 in, 1 out]
        n123 = Bundle By Name(cluster=w162, "时间"=w156, "第一次水样浓度值"=w155) -> (w161:T16)
        n124 = property class="Clust (严格)"(reference=w157) -> (reference out=w158:refnum<vi>, "Value"=w159:T2)  [unwired: 1 in, 1 out]
        n125 = Bundle By Name(cluster=w159, "时间"=w156, "集成干预测试浓度值"=w155) -> (w160:T2)
        n126 = property class="Clust (严格)"(reference=w164, "Value"=w161) -> ()  [unwired: 1 in, 2 out]
        n127 = property class="Clust (严格)"(reference=w158, "Value"=w160) -> ()  [unwired: 1 in, 2 out]
      }
      frame "获取集成干预前测试数据" {
        n128 = case shown="\"CODMn\"" w220 {
          tunnel: ["" "氨氮" "总磷" "总氮" "CODMn" "CODCr"] -> w219
          frame "null", Default {
          }
          frame "氨氮" {
          }
          frame "总磷" {
          }
          frame "总氮" {
          }
          frame "CODMn" {
          }
          frame "CODCr" {
          }
        }
        n129 = call "启动日志.vi"("日志信息"=w226, "Slave ID"=w220) -> ()  [unwired: 9 in, 1 out]
        n130 = global read "ZK断电保存全局变量.vi" "数据库类型"() -> (w218:T17)
        n131 = call "获取最新一笔数据.vi"("数据库类型"=w218, "table"=w219) -> ("检测值"=w217:cluster{"时间":timestamp, "检测值":dbl})  [unwired: 7 in, 2 out]
        n132 = Unbundle By Name(w217) -> ("时间"=w216:timestamp, "检测值"=w215:dbl)
        n133 = call "Add State to Queue.vi"("State(s) In (\"\")"=w228) -> ("States Out"=w227:string)  [unwired: 14 in]
        n134 = property class="Clust (严格)"(reference=w221) -> (reference out=w222:refnum<vi>, "Value"=w223:T2)  [unwired: 1 in, 1 out]
        n135 = Bundle By Name(cluster=w223, "集成干预前测试时间"=w216, "集成干预前测试浓度值"=w215) -> (w224:T2)
        n136 = property class="Clust (严格)"(reference=w222, "Value"=w224) -> ()  [unwired: 1 in, 2 out]
      }
      frame "获取加标回收测试数据" {
        n137 = case shown="\"CODCr\"" w247 {
          tunnel: [sgl 0.0 ("水样实测值") w270 w274 w278 w282 w286] -> w256
          tunnel: [timestamp(0 s since 1904-01-01) ("加标回收数据时间") w269 w273 w277 w281 w285] -> w253
          frame "null", Default {
          }
          frame "氨氮" {
            w267 = u16 3 items=["总磷"=1, "总氮"=2, "氨氮"=3, "CODMn"=21, "CODcr"=22] ("站号")
            n138 = call-poly "获取测试数据.vi"("站号"=w267) -> ("测量数据区"=w268:T18)  [unwired: 10 in]
            n139 = Unbundle By Name(w268) -> ("加标回收数据时间"=w269:timestamp, "加标回收实测值"=w270:sgl)
          }
          frame "总磷" {
            w271 = u16 1 items=["总磷"=1, "总氮"=2, "氨氮"=3, "CODMn"=21, "CODcr"=22] ("站号")
            n140 = call-poly "获取测试数据.vi"("站号"=w271) -> ("测量数据区"=w272:T18)  [unwired: 10 in]
            n141 = Unbundle By Name(w272) -> ("加标回收数据时间"=w273:timestamp, "加标回收实测值"=w274:sgl)
          }
          frame "总氮" {
            w275 = u16 2 items=["总磷"=1, "总氮"=2, "氨氮"=3, "CODMn"=21, "CODcr"=22] ("站号")
            n142 = call-poly "获取测试数据.vi"("站号"=w275) -> ("测量数据区"=w276:T18)  [unwired: 10 in]
            n143 = Unbundle By Name(w276) -> ("加标回收数据时间"=w277:timestamp, "加标回收实测值"=w278:sgl)
          }
          frame "CODMn" {
            w279 = u16 21 items=["总磷"=1, "总氮"=2, "氨氮"=3, "CODMn"=21, "CODcr"=22] ("站号")
            n144 = call-poly "获取测试数据.vi"("站号"=w279) -> ("测量数据区"=w280:T18)  [unwired: 10 in]
            n145 = Unbundle By Name(w280) -> ("加标回收数据时间"=w281:timestamp, "加标回收实测值"=w282:sgl)
          }
          frame "CODCr" {
            w283 = u16 22 items=["总磷"=1, "总氮"=2, "氨氮"=3, "CODMn"=21, "CODcr"=22] ("站号")
            n146 = call-poly "获取测试数据.vi"("站号"=w283) -> ("测量数据区"=w284:T18)  [unwired: 10 in]
            n147 = Unbundle By Name(w284) -> ("加标回收数据时间"=w285:timestamp, "加标回收实测值"=w286:sgl)
          }
        }
        n148 = Index Array(array=w238, index=10 ("索引")) -> (element=w246:refnum<vi>)
        n149 = local read "加标回收启动时间"() -> (w254:timestamp)
        n150 = property class="DigNum (严格)"(reference=w246) -> (reference out=w244:refnum<vi>, "Value"=w243:u16)  [unwired: 1 in, 1 out]
        n151 = call "启动日志.vi"("日志信息"=w236, "Slave ID"=w247) -> ()  [unwired: 9 in, 1 out]
        n152 = local write "加标回收测试时间"(w253) -> ()
        n153 = Subtract(x=w253, y=w254) -> (x-y=w252:dbl)
        n154 = Increment(x=w243) -> (x+1=w242:u16)
        n155 = Absolute Value(x=w252) -> (abs(x)=w249:dbl)
        n156 = Less?(x=w249, y=300.0) -> (x < y?=w248:bool)
        n157 = property class="DigNum (严格)"(reference=w244, "Value"=w242) -> ()  [unwired: 1 in, 2 out]
        n158 = property class="Clust (严格)"(reference=w260) -> (reference out=w259:refnum<vi>, "Value"=w258:T5)  [unwired: 1 in, 1 out]
        n159 = Less Or Equal?(x=w242, y=u16 5) -> (x <= y?=w240:bool)
        n160 = Bundle By Name(cluster=w258, "加标后水样浓度"=w256) -> (w257:T5)
        n161 = property class="Clust (严格)"(reference=w259, "Value"=w257) -> ()  [unwired: 1 in, 2 out]
        n162 = Select(t=w236, s=w240, f="exit") -> (s? t:f=w237:string)
        n163 = Select(t="", s=w248, f=w237) -> (s? t:f=w250:string)
        n164 = call "Add State to Queue.vi"("State(s) In Front (\"\")"=w250, "State(s) In (\"\")"=w262) -> ("States Out"=w261:string)  [unwired: 13 in]
        n165 = case shown="假" w248 {
          tunnel: w247 -> [w264 _]
          frame False {
            w263 = "获取加标数据异常" ("日志信息")
            n166 = call "启动日志.vi"("日志信息"=w263, "Slave ID"=w264) -> ()  [unwired: 9 in, 1 out]
            n167 = call "报警信息记录.vi"("报警信息"=w263, "Slave ID"=w264) -> ()  [unwired: 9 in, 1 out]
          }
          frame True {
          }
        }
      }
      frame "获取平行样测试数据" {
        n168 = case shown="\"CODCr\"" w301 {
          tunnel: [sgl 0.0 ("水样实测值") w322 w326 w330 w334 w338] -> w309
          tunnel: [timestamp(0 s since 1904-01-01) ("加标回收数据时间") w321 w325 w329 w333 w337] -> w287
          frame "null", Default {
          }
          frame "氨氮" {
            w319 = u16 3 items=["总磷"=1, "总氮"=2, "氨氮"=3, "CODMn"=21, "CODcr"=22] ("站号")
            n169 = call-poly "获取测试数据.vi"("站号"=w319) -> ("测量数据区"=w320:T15)  [unwired: 10 in]
            n170 = Unbundle By Name(w320) -> ("水样数据时间"=w321:timestamp, "水样实测值"=w322:sgl)
          }
          frame "总磷" {
            w323 = u16 1 items=["总磷"=1, "总氮"=2, "氨氮"=3, "CODMn"=21, "CODcr"=22] ("站号")
            n171 = call-poly "获取测试数据.vi"("站号"=w323) -> ("测量数据区"=w324:T15)  [unwired: 10 in]
            n172 = Unbundle By Name(w324) -> ("水样数据时间"=w325:timestamp, "水样实测值"=w326:sgl)
          }
          frame "总氮" {
            w327 = u16 2 items=["总磷"=1, "总氮"=2, "氨氮"=3, "CODMn"=21, "CODcr"=22] ("站号")
            n173 = call-poly "获取测试数据.vi"("站号"=w327) -> ("测量数据区"=w328:T15)  [unwired: 10 in]
            n174 = Unbundle By Name(w328) -> ("水样数据时间"=w329:timestamp, "水样实测值"=w330:sgl)
          }
          frame "CODMn" {
            w331 = u16 21 items=["总磷"=1, "总氮"=2, "氨氮"=3, "CODMn"=21, "CODcr"=22] ("站号")
            n175 = call-poly "获取测试数据.vi"("站号"=w331) -> ("测量数据区"=w332:T15)  [unwired: 10 in]
            n176 = Unbundle By Name(w332) -> ("水样数据时间"=w333:timestamp, "水样实测值"=w334:sgl)
          }
          frame "CODCr" {
            w335 = u16 22 items=["总磷"=1, "总氮"=2, "氨氮"=3, "CODMn"=21, "CODcr"=22] ("站号")
            n177 = call-poly "获取测试数据.vi"("站号"=w335) -> ("测量数据区"=w336:T15)  [unwired: 10 in]
            n178 = Unbundle By Name(w336) -> ("水样数据时间"=w337:timestamp, "水样实测值"=w338:sgl)
          }
        }
        n179 = Index Array(array=w292, index=10 ("索引")) -> (element=w300:refnum<vi>)
        n180 = property class="DigNum (严格)"(reference=w300) -> (reference out=w298:refnum<vi>, "Value"=w297:u16)  [unwired: 1 in, 1 out]
        n181 = local read "平行样启动时间"() -> (w307:timestamp)
        n182 = call "启动日志.vi"("日志信息"=w290, "Slave ID"=w301) -> ()  [unwired: 9 in, 1 out]
        n183 = Subtract(x=w287, y=w307) -> (x-y=w306:dbl)
        n184 = Increment(x=w297) -> (x+1=w296:u16)
        n185 = Absolute Value(x=w306) -> (abs(x)=w303:dbl)
        n186 = Less?(x=w303, y=300.0) -> (x < y?=w302:bool)
        n187 = property class="DigNum (严格)"(reference=w298, "Value"=w296) -> ()  [unwired: 1 in, 2 out]
        n188 = property class="Clust (严格)"(reference=w288) -> (reference out=w312:refnum<vi>, "Value"=w311:T16)  [unwired: 1 in, 1 out]
        n189 = Less Or Equal?(x=w296, y=u16 5) -> (x <= y?=w294:bool)
        n190 = Bundle By Name(cluster=w311, "第二次水样测试时间"=w287, "第二次水样浓度值"=w309) -> (w310:T16)
        n191 = property class="Clust (严格)"(reference=w312, "Value"=w310) -> ()  [unwired: 1 in, 2 out]
        n192 = Select(t=w290, s=w294, f="exit") -> (s? t:f=w291:string)
        n193 = Select(t="", s=w302, f=w291) -> (s? t:f=w304:string)
        n194 = call "Add State to Queue.vi"("State(s) In Front (\"\")"=w304, "State(s) In (\"\")"=w314) -> ("States Out"=w313:string)  [unwired: 13 in]
        n195 = case shown="假" w302 {
          tunnel: w301 -> [w316 _]
          frame False {
            w315 = "获取平行样数据异常" ("日志信息")
            n196 = call "启动日志.vi"("日志信息"=w315, "Slave ID"=w316) -> ()  [unwired: 9 in, 1 out]
            n197 = call "报警信息记录.vi"("报警信息"=w315, "Slave ID"=w316) -> ()  [unwired: 9 in, 1 out]
          }
          frame True {
          }
        }
      }
      frame "计算加标体积" {
        n198 = call "启动日志.vi"("日志信息"=w341, "Slave ID"=w340) -> ()  [unwired: 9 in, 1 out]
        n199 = property class="Clust (严格)"(reference=w347) -> (reference out=w346:refnum<vi>, "Value"=w345:T5)  [unwired: 1 in, 1 out]
        n200 = call "加标回收率计算.vi"("参数"=w345) -> ("参数 out"=w344:T5)  [unwired: 9 in, 1 out]
        n201 = Bundle By Name(cluster=w344, "加标回收率"=0.0) -> (w343:T5)
        n202 = property class="Clust (严格)"(reference=w346, "Value"=w343) -> ()  [unwired: 1 in, 2 out]
        n203 = call "Add State to Queue.vi"("State(s) In (\"\")"=w349) -> ("States Out"=w348:string)  [unwired: 14 in]
      }
      frame "计算加标回收率" {
        n204 = call "启动日志.vi"("日志信息"=w351, "Slave ID"=w352) -> ()  [unwired: 9 in, 1 out]
        n205 = property class="Clust (严格)"(reference=w356) -> (reference out=w355:refnum<vi>, "Value"=w354:T5)  [unwired: 1 in, 1 out]
        n206 = call "加标回收率计算.vi"("参数"=w354) -> ("参数 out"=w353:T5)  [unwired: 9 in, 1 out]
        n207 = property class="Clust (严格)"(reference=w355, "Value"=w353) -> ()  [unwired: 1 in, 2 out]
        n208 = call "Add State to Queue.vi"("State(s) In (\"\")"=w358) -> ("States Out"=w357:string)  [unwired: 14 in]
      }
      frame "存储加标回收测试数据" {
        n209 = case shown="\"总氮\"" w363 {
          tunnel: ["" "氨氮加标回收率" "总磷加标回收率" "总氮加标回收率" "CODMn加标回收率" "CODCr加标回收率"] -> w364
          frame "null", Default {
          }
          frame "氨氮" {
          }
          frame "总磷" {
          }
          frame "总氮" {
          }
          frame "CODMn" {
          }
          frame "CODCr" {
          }
        }
        n210 = property class="Clust (严格)"(reference=w374) -> ("Value"=w371:T5)  [unwired: 1 in, 2 out]
        n211 = Unbundle By Name(w371) -> ("加标前水样浓度"=w370:dbl, "加标后水样浓度"=w369:dbl, "加标母液浓度"=w368:dbl, "加标体积"=w367:dbl, "加标水杯定容体积"=w366:dbl, "加标回收率"=w365:dbl)
        n212 = call "启动日志.vi"("日志信息"=w362, "Slave ID"=w363) -> ()  [unwired: 9 in, 1 out]
        n213 = Bundle By Name(cluster=T8 {"时间"=timestamp(0 s since 1904-01-01), "参数"="", "数据类型"="N", "加标回收率"=0.0, "加标前水样测试时间"=timestamp(0 s since 1904-01-01), "加标前水样浓度值"=0.0, "加标后水样浓度值"=0.0, "加标母液浓度值"=0.0, "加标体积"=0.0, "加标水杯定容体积"=0.0} ("data in"), "时间"="加标回收测试时间", "参数"=w364, "加标前水样测试时间"="水样测试时间", "加标前水样浓度值"=w370, "加标后水样浓度值"=w369, "加标母液浓度值"=w368, "加标体积"=w367, "加标水杯定容体积"=w366, "加标回收率"=w365) -> (w360:T8)
        n214 = call "加标回收数据插入.vi"("data in"=w360) -> ()  [unwired: 10 in, 1 out]
        n215 = call "Add State to Queue.vi"("State(s) In (\"\")"=w376) -> ("States Out"=w375:string)  [unwired: 14 in]
      }
      frame "存储平行样测试数据" {
        n216 = case shown="\"CODMn\"" w390 {
          tunnel: ["" "氨氮" "总磷" "总氮" "CODMn" "CODCr"] -> w383
          frame "null", Default {
          }
          frame "氨氮" {
          }
          frame "总磷" {
          }
          frame "总氮" {
          }
          frame "CODMn" {
          }
          frame "CODCr" {
          }
        }
        n217 = property class="Clust (严格)"(reference=w387) -> (reference out=w385:refnum<vi>, "Value"=w386:T16)  [unwired: 1 in, 1 out]
        n218 = Bundle By Name(cluster=w386, "参数"=w383) -> (w384:T16)
        n219 = call "启动日志.vi"("日志信息"=w389, "Slave ID"=w390) -> ()  [unwired: 9 in, 1 out]
        n220 = property class="Clust (严格)"(reference=w385, "Value"=w384) -> ()  [unwired: 1 in, 2 out]
        n221 = call "平行样数据插入.vi"("平行样测试数据"=w384) -> ()  [unwired: 10 in, 1 out]
        n222 = call "Add State to Queue.vi"("State(s) In (\"\")"=w392) -> ("States Out"=w391:string)  [unwired: 14 in]
      }
      frame "存储集成干预测试数据" {
        n223 = property class="Clust (严格)"(reference=w404) -> (reference out=w402:refnum<vi>, "Value"=w403:T2)  [unwired: 1 in, 1 out]
        n224 = case shown="\"CODMn\"" w401 {
          tunnel: ["" "氨氮" "总磷" "总氮" "CODMn" "CODCr"] -> w400
          frame "null", Default {
          }
          frame "氨氮" {
          }
          frame "总磷" {
          }
          frame "总氮" {
          }
          frame "CODMn" {
          }
          frame "CODCr" {
          }
        }
        n225 = Bundle By Name(cluster=w403, "参数"=w400) -> (w399:T2)
        n226 = call "启动日志.vi"("日志信息"=w406, "Slave ID"=w401) -> ()  [unwired: 9 in, 1 out]
        n227 = property class="Clust (严格)"(reference=w402, "Value"=w399) -> ()  [unwired: 1 in, 2 out]
        n228 = call "集成干预数据插入.vi"("集成干预测试数据"=w399) -> ()  [unwired: 10 in, 1 out]
        n229 = call "Add State to Queue.vi"("State(s) In (\"\")"=w408) -> ("States Out"=w407:string)  [unwired: 14 in]
      }
      frame "流程结束" {
        n230 = Concatenate Strings("----->>" ("字符串"), w418) -> (w417:string)
        n231 = call "启动日志.vi"("日志信息"=w417, "Slave ID"=w419) -> ()  [unwired: 9 in, 1 out]
        n232 = global read "ZK非断电保存全局变量.vi" "流程运行状态标记位"() -> (w421:T7)
        n233 = case shown="\"CODCr\"" w419 {
          tunnel: "空闲" -> [_ w425 w426 w427 w428 w429]
          frame "null", Default {
          }
          frame "氨氮" {
            n234 = global write "ZK非断电保存全局变量.vi" "氨氮加标模块运行状态"(w425) -> ()
          }
          frame "总磷" {
            n235 = global write "ZK非断电保存全局变量.vi" "总磷加标模块运行状态"(w426) -> ()
          }
          frame "总氮" {
            n236 = global write "ZK非断电保存全局变量.vi" "总氮加标模块运行状态"(w427) -> ()
          }
          frame "CODMn" {
            n237 = global write "ZK非断电保存全局变量.vi" "CODMn加标模块运行状态"(w428) -> ()
          }
          frame "CODCr" {
            n238 = global write "ZK非断电保存全局变量.vi" "CODcr加标模块运行状态"(w429) -> ()
          }
        }
        n239 = case shown="\"总磷\"" w419 {
          tunnel: w421 -> [_ w432 w433 w436 w439 w442]
          frame "null", Default {
          }
          frame "氨氮" {
            n240 = Bundle By Name(cluster=w432, "氨氮"=FALSE) -> (w431:T7)
            n241 = global write "ZK非断电保存全局变量.vi" "流程运行状态标记位"(w431) -> ()
          }
          frame "总磷" {
            n242 = Bundle By Name(cluster=w433, "总磷"=FALSE ("氨氮")) -> (w435:T7)
            n243 = global write "ZK非断电保存全局变量.vi" "流程运行状态标记位"(w435) -> ()
          }
          frame "总氮" {
            n244 = Bundle By Name(cluster=w436, "总氮"=FALSE ("氨氮")) -> (w438:T7)
            n245 = global write "ZK非断电保存全局变量.vi" "流程运行状态标记位"(w438) -> ()
          }
          frame "CODMn" {
            n246 = Bundle By Name(cluster=w439, "CODMn"=FALSE ("氨氮")) -> (w441:T7)
            n247 = global write "ZK非断电保存全局变量.vi" "流程运行状态标记位"(w441) -> ()
          }
          frame "CODCr" {
            n248 = Bundle By Name(cluster=w442, "CODCr"=FALSE ("氨氮")) -> (w444:T7)
            n249 = global write "ZK非断电保存全局变量.vi" "流程运行状态标记位"(w444) -> ()
          }
        }
        n250 = call "Add State to Queue.vi"("State(s) In (\"\")"=w424) -> ("States Out"=w423:string)  [unwired: 14 in]
      }
      frame "流程退出" {
        n251 = Concatenate Strings("----->>" ("字符串"), w448) -> (w447:string)
        n252 = call "启动日志.vi"("日志信息"=w447, "Slave ID"=w449) -> ()  [unwired: 9 in, 1 out]
        n253 = call "Add State to Queue.vi"("State(s) In (\"\")"=w452) -> ("States Out"=w451:string)  [unwired: 14 in]
      }
      frame "-------------------# 采配水流程 #-------------------" {
        n254 = call "Add State to Queue.vi"("State(s) In (\"\")"=w455) -> ("States Out"=w454:string)  [unwired: 14 in]
      }
      frame "采水单元启动水样测试流程" {
        n255 = Index Array(array=w464) -> (element=w463:refnum<vi>)  [unwired: 1 in]
        n256 = property class="DigNum (严格)"(reference=w463) -> (reference out=w462:refnum<vi>, "Value"=w461:u16)  [unwired: 1 in, 1 out]
        n257 = call "启动日志.vi"("日志信息"=w458, "Slave ID"=w459) -> ()  [unwired: 9 in, 1 out]
        n258 = Increment(x=w461) -> (x+1=w460:u16)
        n259 = property class="DigNum (严格)"(reference=w462, "Value"=w460) -> ()  [unwired: 1 in, 2 out]
        n260 = call "采配水启动器.vi"("启动/停止命令"=T9."水样测试（全流程）") -> ()  [unwired: 10 in, 1 out]
        n261 = call "Add State to Queue.vi"("State(s) In (\"\")"=w466) -> ("States Out"=w465:string)  [unwired: 14 in]
      }
      frame "采水单元启动加标回收流程" {
        n262 = Index Array(array=w475) -> (element=w474:refnum<vi>)  [unwired: 1 in]
        n263 = call "启动日志.vi"("日志信息"=w469, "Slave ID"=w470) -> ()  [unwired: 9 in, 1 out]
        n264 = property class="DigNum (严格)"(reference=w474) -> (reference out=w473:refnum<vi>, "Value"=w472:u16)  [unwired: 1 in, 1 out]
        n265 = Increment(x=w472) -> (x+1=w471:u16)
        n266 = property class="DigNum (严格)"(reference=w473, "Value"=w471) -> ()  [unwired: 1 in, 2 out]
        n267 = call "采配水启动器.vi"("启动/停止命令"=T9."加标回收") -> ()  [unwired: 10 in, 1 out]
        n268 = call "Add State to Queue.vi"("State(s) In (\"\")"=w477) -> ("States Out"=w476:string)  [unwired: 14 in]
      }
      frame "判断采水单元水样测试流程是否启动" {
        n269 = Index Array(array=w485, index=0 ("索引")) -> (element=w484:refnum<vi>)
        n270 = property class="DigNum (严格)"(reference=w484) -> ("Value"=w483:u16)  [unwired: 1 in, 2 out]
        n271 = call "获取采配水运行状态.vi"() -> ("运行流程"=w494:T11)  [unwired: 10 in, 1 out]
        n272 = call "启动日志.vi"("日志信息"=w481, "Slave ID"=w480) -> ()  [unwired: 9 in, 1 out]
        n273 = Equal?(x=T10."待机" ("运行流程"), y=w494) -> (x = y?=w493:bool)
        n274 = Select(t="采水单元启动水样测试流程\n判断采水单元水样测试流程是否启动" ("State(s) In (\"\")"), s=w493, f="") -> (s? t:f=w488:string)
        n275 = Greater Or Equal?(x=w483, y=u16 5) -> (x >= y?=w479:bool)
        n276 = case shown="真" w479 {
          tunnel: w480 -> [_ w498]
          frame False {
          }
          frame True {
            w497 = "采水单元启动失败" ("日志信息")
            n277 = call "启动日志.vi"("日志信息"=w497, "Slave ID"=w498) -> ()  [unwired: 9 in, 1 out]
            n278 = call "报警信息记录.vi"("报警信息"=w497, "Slave ID"=w498) -> ()  [unwired: 9 in, 1 out]
          }
        }
        n279 = Select(t="流程结束" ("State(s) In (\"\")"), s=w479, f=w488) -> (s? t:f=w487:string)
        n280 = call "Add State to Queue.vi"("State(s) In Front (\"\")"=w487, "State(s) In (\"\")"=w496) -> ("States Out"=w495:string)  [unwired: 13 in]
      }
      frame "判断采水单元加标回收流程是否启动" {
        n281 = Index Array(array=w507, index=0 ("索引")) -> (element=w506:refnum<vi>)
        n282 = property class="DigNum (严格)"(reference=w506) -> ("Value"=w505:u16)  [unwired: 1 in, 2 out]
        n283 = call "获取采配水运行状态.vi"() -> ("运行流程"=w516:T11)  [unwired: 10 in, 1 out]
        n284 = call "启动日志.vi"("日志信息"=w502, "Slave ID"=w501) -> ()  [unwired: 9 in, 1 out]
        n285 = Equal?(x=T10."待机" ("运行流程"), y=w516) -> (x = y?=w515:bool)
        n286 = Select(t="采水单元启动加标回收流程\n判断采水单元加标回收流程是否启动" ("State(s) In (\"\")"), s=w515, f="") -> (s? t:f=w510:string)
        n287 = Greater Or Equal?(x=w505, y=u16 5) -> (x >= y?=w500:bool)
        n288 = case shown="真" w500 {
          tunnel: w501 -> [_ w519]
          frame False {
          }
          frame True {
            w518 = "采水单元启动失败" ("日志信息")
            n289 = call "启动日志.vi"("日志信息"=w518, "Slave ID"=w519) -> ()  [unwired: 9 in, 1 out]
            n290 = call "报警信息记录.vi"("报警信息"=w518, "Slave ID"=w519) -> ()  [unwired: 9 in, 1 out]
          }
        }
        n291 = Select(t="流程结束" ("State(s) In (\"\")"), s=w500, f=w510) -> (s? t:f=w509:string)
        n292 = call "Add State to Queue.vi"("State(s) In Front (\"\")"=w509, "State(s) In (\"\")"=w503) -> ("States Out"=w517:string)  [unwired: 13 in]
      }
      frame "采水单元润洗" {
        n293 = call "获取采配水运行状态.vi"() -> ("运行流程"=w530:T11)  [unwired: 10 in, 1 out]
        n294 = case shown="真" w520 {
          tunnel: w523 -> [_ w540]
          tunnel: w524 -> [_ w539]
          frame False {
          }
          frame True {
            n295 = call "启动日志.vi"("日志信息"=w539, "Slave ID"=w540) -> ()  [unwired: 9 in, 1 out]
          }
        }
        n296 = Less?(x=w530, y=T10."采样" ("运行流程")) -> (x < y?=w533:bool)
        n297 = Greater?(x=w530, y=T10."待机" ("运行流程")) -> (0:w534:bool)
        n298 = And(x=w533, y=w534) -> (x .and. y?=w532:bool)
        n299 = Select(t=w524, s=w532, f="") -> (s? t:f=w528:string)
        n300 = Equal To 0?(x=w530) -> (x = 0?=w522:bool)
        n301 = case shown="真" w522 {
          tunnel: w523 -> [_ w538]
          frame False {
          }
          frame True {
            w537 = "采水单元流程中断" ("日志信息")
            n302 = call "启动日志.vi"("日志信息"=w537, "Slave ID"=w538) -> ()  [unwired: 9 in, 1 out]
            n303 = call "报警信息记录.vi"("报警信息"=w537, "Slave ID"=w538) -> ()  [unwired: 9 in, 1 out]
          }
        }
        n304 = Select(t="流程结束" ("State(s) In (\"\")"), s=w522, f=w528) -> (s? t:f=w527:string)
        n305 = call "Add State to Queue.vi"("State(s) In Front (\"\")"=w527, "State(s) In (\"\")"=w536) -> ("States Out"=w535:string)  [unwired: 13 in]
      }
      frame "采水单元采样" {
        n306 = call "获取采配水运行状态.vi"() -> ("运行流程"=w547:T11)  [unwired: 10 in, 1 out]
        n307 = case shown="真" w541 {
          tunnel: w543 -> [_ w558]
          tunnel: w545 -> [_ w557]
          frame False {
          }
          frame True {
            n308 = call "启动日志.vi"("日志信息"=w557, "Slave ID"=w558) -> ()  [unwired: 9 in, 1 out]
          }
        }
        n309 = Equal?(x=T10."采样" ("运行流程"), y=w547) -> (x = y?=w546:bool)
        n310 = Select(t=w545, s=w546, f="") -> (s? t:f=w550:string)
        n311 = Equal To 0?(x=w547) -> (x = 0?=w544:bool)
        n312 = case shown="真" w544 {
          tunnel: w543 -> [_ w556]
          frame False {
          }
          frame True {
            w555 = "采水单元流程中断" ("日志信息")
            n313 = call "启动日志.vi"("日志信息"=w555, "Slave ID"=w556) -> ()  [unwired: 9 in, 1 out]
            n314 = call "报警信息记录.vi"("报警信息"=w555, "Slave ID"=w556) -> ()  [unwired: 9 in, 1 out]
          }
        }
        n315 = Select(t="流程结束" ("State(s) In (\"\")"), s=w544, f=w550) -> (s? t:f=w549:string)
        n316 = call "Add State to Queue.vi"("State(s) In Front (\"\")"=w549, "State(s) In (\"\")"=w554) -> ("States Out"=w553:string)  [unwired: 13 in]
      }
      frame "水样沉淀" {
        n317 = global read "系统交互.vi" "站点类型"() -> (w564:enum16{"一体站", "固定站", "浮船"})
        n318 = case shown="\"浮船\"" w564 {
          tunnel: [w578 _ _] -> w565
          tunnel: w560 -> [w577 _ _]
          frame "一体站", Default {
            n319 = case shown="真" w577 {
              tunnel: [_ w579] -> w578
              frame False {
              }
              frame True {
                n320 = call "质控模块润洗OK命令.vi"("质控润洗OK"=TRUE) -> ("error out"=w579:errorcluster)  [unwired: 10 in]
              }
            }
          }
          frame "固定站" {
          }
          frame "浮船" {
          }
        }
        n321 = case shown="真" w560 {
          tunnel: w563 -> [_ w582]
          tunnel: w566 -> [_ w581]
          frame False {
          }
          frame True {
            n322 = call "启动日志.vi"("日志信息"=w581, "Slave ID"=w582) -> ()  [unwired: 9 in, 1 out]
          }
        }
        n323 = call "获取采配水运行状态.vi"("error in (no error)"=w565) -> ("运行流程"=w570:T11)  [unwired: 9 in, 1 out]
        n324 = Equal?(x=采配水通用流程."沉淀" ("运行流程"), y=w570) -> (x = y?=w572:bool)
        n325 = Equal To 0?(x=w570) -> (x = 0?=w562:bool)
        n326 = Select(t=w566, s=w572, f="") -> (s? t:f=w568:string)
        n327 = case shown="真" w562 {
          tunnel: w563 -> [_ w576]
          frame False {
          }
          frame True {
            w575 = "采水单元流程中断" ("日志信息")
            n328 = call "启动日志.vi"("日志信息"=w575, "Slave ID"=w576) -> ()  [unwired: 9 in, 1 out]
            n329 = call "报警信息记录.vi"("报警信息"=w575, "Slave ID"=w576) -> ()  [unwired: 9 in, 1 out]
          }
        }
        n330 = Select(t="流程结束" ("State(s) In (\"\")"), s=w562, f=w568) -> (s? t:f=w567:string)
        n331 = call "Add State to Queue.vi"("State(s) In Front (\"\")"=w567, "State(s) In (\"\")"=w574) -> ("States Out"=w573:string)  [unwired: 13 in]
      }
      frame "水样配水" {
        n332 = call "获取采配水运行状态.vi"() -> ("运行流程"=w593:T11)  [unwired: 10 in, 1 out]
        n333 = case shown="真" w584 {
          tunnel: w586 -> [_ w600]
          tunnel: w588 -> [_ w599]
          frame False {
          }
          frame True {
            n334 = call "启动日志.vi"("日志信息"=w599, "Slave ID"=w600) -> ()  [unwired: 9 in, 1 out]
          }
        }
        n335 = Equal?(x=采配水通用流程."配水" ("运行流程"), y=w593) -> (x = y?=w594:bool)
        n336 = Equal To 0?(x=w593) -> (x = 0?=w587:bool)
        n337 = Select(t="", s=w594, f=w588) -> (s? t:f=w591:string)
        n338 = case shown="真" w587 {
          tunnel: w586 -> [_ w598]
          frame False {
          }
          frame True {
            w597 = "采水单元流程中断" ("日志信息")
            n339 = call "启动日志.vi"("日志信息"=w597, "Slave ID"=w598) -> ()  [unwired: 9 in, 1 out]
            n340 = call "报警信息记录.vi"("报警信息"=w597, "Slave ID"=w598) -> ()  [unwired: 9 in, 1 out]
          }
        }
        n341 = Select(t="流程结束" ("State(s) In (\"\")"), s=w587, f=w591) -> (s? t:f=w590:string)
        n342 = call "Add State to Queue.vi"("State(s) In Front (\"\")"=w590, "State(s) In (\"\")"=w596) -> ("States Out"=w595:string)  [unwired: 13 in]
      }
      frame "-------------------# 质控模块流程 #-------------------" {
        n343 = call "Add State to Queue.vi"("State(s) In (\"\")"=w603) -> ("States Out"=w602:string)  [unwired: 14 in]
      }
      frame "质控单元启动水样润洗" {
        w613 = 质控流程控制."启动水样润洗流程" ("流程控制")
        n344 = Index Array(array=w608, index=1 ("索引")) -> (element=w612:refnum<vi>)
        n345 = property class="DigNum (严格)"(reference=w612) -> (reference out=w611:refnum<vi>, "Value"=w610:u16)  [unwired: 1 in, 1 out]
        n346 = call "ZK流程控制.vi"("流程控制"=w613, "Slave ID"=w606) -> ()  [unwired: 9 in, 1 out]
        n347 = Increment(x=w610) -> (x+1=w609:u16)
        n348 = property class="DigNum (严格)"(reference=w611, "Value"=w609) -> ()  [unwired: 1 in, 2 out]
        n349 = call "启动日志.vi"("日志信息"=w605, "Slave ID"=w606) -> ()  [unwired: 9 in, 1 out]
        n350 = call "Add State to Queue.vi"("State(s) In (\"\")"=w615) -> ("States Out"=w614:string)  [unwired: 14 in]
        "加标模块润洗流程控制" <- w613
      }
      frame "质控单元启动加标润洗" {
        w617 = 质控流程控制."启动加标润洗流程" ("流程控制")
        n351 = Index Array(array=w621, index=7 ("索引")) -> (element=w625:refnum<vi>)
        n352 = property class="DigNum (严格)"(reference=w625) -> (reference out=w624:refnum<vi>, "Value"=w623:u16)  [unwired: 1 in, 1 out]
        n353 = local write "加标模块润洗流程控制"(w617) -> ()
        n354 = call "ZK流程控制.vi"("流程控制"=w617, "Slave ID"=w619) -> ()  [unwired: 9 in, 1 out]
        n355 = Increment(x=w623) -> (x+1=w622:u16)
        n356 = property class="DigNum (严格)"(reference=w624, "Value"=w622) -> ()  [unwired: 1 in, 2 out]
        n357 = call "启动日志.vi"("日志信息"=w618, "Slave ID"=w619) -> ()  [unwired: 9 in, 1 out]
        n358 = call "Add State to Queue.vi"("State(s) In (\"\")"=w627) -> ("States Out"=w626:string)  [unwired: 14 in]
      }
      frame "质控单元启动采样" {
        n359 = Index Array(array=w632, index=2 ("索引")) -> (element=w636:refnum<vi>)
        n360 = call "ZK流程控制.vi"("流程控制"=质控流程控制."启动进样流程", "Slave ID"=w630) -> ()  [unwired: 9 in, 1 out]
        n361 = property class="DigNum (严格)"(reference=w636) -> (reference out=w635:refnum<vi>, "Value"=w634:u16)  [unwired: 1 in, 1 out]
        n362 = Increment(x=w634) -> (x+1=w633:u16)
        n363 = property class="DigNum (严格)"(reference=w635, "Value"=w633) -> ()  [unwired: 1 in, 2 out]
        n364 = call "启动日志.vi"("日志信息"=w629, "Slave ID"=w630) -> ()  [unwired: 9 in, 1 out]
        n365 = call "Add State to Queue.vi"("State(s) In (\"\")"=w639) -> ("States Out"=w638:string)  [unwired: 14 in]
      }
      frame "质控单元写入加标体积" {
        n366 = Index Array(array=w646, index=8 ("索引")) -> (element=w644:refnum<vi>)
        n367 = property class="Clust (严格)"(reference=w652) -> ("Value"=w651:T5)  [unwired: 1 in, 2 out]
        n368 = property class="DigNum (严格)"(reference=w644) -> (reference out=w642:refnum<vi>, "Value"=w643:u16)  [unwired: 1 in, 1 out]
        n369 = Unbundle By Name(w651) -> ("加标体积"=w650:dbl)
        n370 = call "启动日志.vi"("日志信息"=w647, "Slave ID"=w641) -> ()  [unwired: 9 in, 1 out]
        n371 = call "ZK加标体积写入.vi"("加标体积"=w650, "Slave ID"=w641) -> ("error out"=w649:errorcluster)  [unwired: 9 in]
        n372 = case shown="错误" w649 {
          tunnel: [_ w657] -> w648
          tunnel: w647 -> [_ w659]
          tunnel: w643 -> [_ w661]
          tunnel: w642 -> [_ w663]
          tunnel: w641 -> [_ w655]
          frame No Error {
          }
          frame Error {
            n373 = Greater Or Equal?(x=w661, y=u16 5) -> (x >= y?=w656:bool)
            n374 = Increment(x=w661) -> (x+1=w662:u16)
            n375 = case shown="真" w656 {
              tunnel: w655 -> [_ w665]
              frame False {
              }
              frame True {
                w664 = "加标体积写入异常" ("报警信息")
                n376 = call "启动日志.vi"("日志信息"=w664, "Slave ID"=w665) -> ()  [unwired: 9 in, 1 out]
                n377 = call "报警信息记录.vi"("报警信息"=w664, "Slave ID"=w665) -> ()  [unwired: 9 in, 1 out]
              }
            }
            n378 = property class="DigNum (严格)"(reference=w663, "Value"=w662) -> ()  [unwired: 1 in, 2 out]
            n379 = Select(t="流程结束", s=w656, f=w659) -> (s? t:f=w657:string)
          }
        }
        n380 = call "Add State to Queue.vi"("State(s) In Front (\"\")"=w648, "State(s) In (\"\")"=w654) -> ("States Out"=w653:string)  [unwired: 13 in]
      }
      frame "质控单元启动加标" {
        n381 = Index Array(array=w671, index=3 ("索引")) -> (element=w670:refnum<vi>)
        n382 = call "ZK流程控制.vi"("流程控制"=质控流程控制."启动加标流程", "Slave ID"=w668) -> ()  [unwired: 9 in, 1 out]
        n383 = property class="DigNum (严格)"(reference=w670) -> (reference out=w674:refnum<vi>, "Value"=w673:u16)  [unwired: 1 in, 1 out]
        n384 = call "启动日志.vi"("日志信息"=w667, "Slave ID"=w668) -> ()  [unwired: 9 in, 1 out]
        n385 = Increment(x=w673) -> (x+1=w672:u16)
        n386 = property class="DigNum (严格)"(reference=w674, "Value"=w672) -> ()  [unwired: 1 in, 2 out]
        n387 = call "Add State to Queue.vi"("State(s) In (\"\")"=w677) -> ("States Out"=w676:string)  [unwired: 14 in]
      }
      frame "质控单元启动排液" {
        n388 = Index Array(array=w683, index=4 ("索引")) -> (element=w682:refnum<vi>)
        n389 = property class="DigNum (严格)"(reference=w682) -> (reference out=w686:refnum<vi>, "Value"=w685:u16)  [unwired: 1 in, 1 out]
        n390 = call "ZK流程控制.vi"("流程控制"=质控流程控制."启动排液流程", "Slave ID"=w680) -> ()  [unwired: 9 in, 1 out]
        n391 = call "启动日志.vi"("日志信息"=w679, "Slave ID"=w680) -> ()  [unwired: 9 in, 1 out]
        n392 = Increment(x=w685) -> (x+1=w684:u16)
        n393 = property class="DigNum (严格)"(reference=w686, "Value"=w684) -> ()  [unwired: 1 in, 2 out]
        n394 = call "Add State to Queue.vi"("State(s) In (\"\")"=w689) -> ("States Out"=w688:string)  [unwired: 14 in]
      }
      frame "质控单元启动搅拌" {
        n395 = call "启动日志.vi"("日志信息"=w694, "Slave ID"=w691) -> ()  [unwired: 9 in, 1 out]
        n396 = call "ZK组合命令区.vi"("是否启用通讯通知"=FALSE, "组合命令区"=质控组合命令区."进空气（搅拌）", "Slave ID"=w691) -> ()  [unwired: 8 in, 1 out]
        n397 = call "Add State to Queue.vi"("State(s) In (\"\")"=w696) -> ("States Out"=w695:string)  [unwired: 14 in]
      }
      frame "判断质控单元润洗是否启动成功" {
        n398 = local read "加标模块润洗流程控制"() -> (w699:T3)
        n399 = Index Array(array=w706, index=1 ("索引")) -> (element=w705:refnum<vi>)
        n400 = case shown="\"CODCr\"" w700 {
          tunnel: [T13."待机" ("运行状态") w722 w724 w726 w728 w730] -> w713
          frame "null", Default {
          }
          frame "氨氮" {
            n401 = global read "ZK非断电保存全局变量.vi" "氨氮质控仪器状态"() -> (w723:T19)
            n402 = Unbundle By Name(w723) -> ("运行状态"=w722:T13)
          }
          frame "总磷" {
            n403 = global read "ZK非断电保存全局变量.vi" "总磷质控仪器状态"() -> (w725:T19)
            n404 = Unbundle By Name(w725) -> ("运行状态"=w724:T13)
          }
          frame "总氮" {
            n405 = global read "ZK非断电保存全局变量.vi" "总氮质控仪器状态"() -> (w727:T19)
            n406 = Unbundle By Name(w727) -> ("运行状态"=w726:T13)
          }
          frame "CODMn" {
            n407 = global read "ZK非断电保存全局变量.vi" "CODMn质控仪器状态"() -> (w729:T19)
            n408 = Unbundle By Name(w729) -> ("运行状态"=w728:T13)
          }
          frame "CODCr" {
            n409 = global read "ZK非断电保存全局变量.vi" "CODCr质控仪器状态"() -> (w731:T19)
            n410 = Unbundle By Name(w731) -> ("运行状态"=w730:T13)
          }
        }
        n411 = property class="DigNum (严格)"(reference=w705) -> ("Value"=w704:u16)  [unwired: 1 in, 2 out]
        n412 = case shown="\"启动加标润洗流程\"" w699 {
          tunnel: ["质控单元启动水样润洗\n判断质控单元润洗是否启动成功" ("State(s) In (\"\")") "质控单元启动加标润洗\n判断质控单元润洗是否启动成功" ("State(s) In (\"\")")] -> w698
          frame "启动水样润洗流程", Default {
          }
          frame "启动加标润洗流程" {
          }
        }
        n413 = call "启动日志.vi"("日志信息"=w702, "Slave ID"=w700) -> ()  [unwired: 9 in, 1 out]
        n414 = Not Equal?(x=w713, y=T13."待机") -> (x != y?=w712:bool)
        n415 = Greater Or Equal?(x=w704, y=u16 5) -> (x >= y?=w701:bool)
        n416 = Select(t="", s=w712, f=w698) -> (s? t:f=w710:string)
        n417 = Select(t="流程结束" ("State(s) In (\"\")"), s=w701, f=w710) -> (s? t:f=w708:string)
        n418 = case shown="真" w701 {
          tunnel: w700 -> [_ w720]
          frame False {
          }
          frame True {
            w719 = "质控单元润洗启动失败" ("日志信息")
            n419 = call "启动日志.vi"("日志信息"=w719, "Slave ID"=w720) -> ()  [unwired: 9 in, 1 out]
            n420 = call "报警信息记录.vi"("报警信息"=w719, "Slave ID"=w720) -> ()  [unwired: 9 in, 1 out]
          }
        }
        n421 = call "Add State to Queue.vi"("State(s) In Front (\"\")"=w708, "State(s) In (\"\")"=w716) -> ("States Out"=w715:string)  [unwired: 13 in]
      }
      frame "判断质控单元采样是否启动成功" {
        n422 = case shown="\"CODCr\"" w733 {
          tunnel: [T13."待机" ("运行状态") w754 w756 w758 w760 w762] -> w747
          frame "null", Default {
          }
          frame "氨氮" {
            n423 = global read "ZK非断电保存全局变量.vi" "氨氮质控仪器状态"() -> (w755:T19)
            n424 = Unbundle By Name(w755) -> ("运行状态"=w754:T13)
          }
          frame "总磷" {
            n425 = global read "ZK非断电保存全局变量.vi" "总磷质控仪器状态"() -> (w757:T19)
            n426 = Unbundle By Name(w757) -> ("运行状态"=w756:T13)
          }
          frame "总氮" {
            n427 = global read "ZK非断电保存全局变量.vi" "总氮质控仪器状态"() -> (w759:T19)
            n428 = Unbundle By Name(w759) -> ("运行状态"=w758:T13)
          }
          frame "CODMn" {
            n429 = global read "ZK非断电保存全局变量.vi" "CODMn质控仪器状态"() -> (w761:T19)
            n430 = Unbundle By Name(w761) -> ("运行状态"=w760:T13)
          }
          frame "CODCr" {
            n431 = global read "ZK非断电保存全局变量.vi" "CODCr质控仪器状态"() -> (w763:T19)
            n432 = Unbundle By Name(w763) -> ("运行状态"=w762:T13)
          }
        }
        n433 = Index Array(array=w739, index=2 ("索引")) -> (element=w738:refnum<vi>)
        n434 = call "启动日志.vi"("日志信息"=w735, "Slave ID"=w733) -> ()  [unwired: 9 in, 1 out]
        n435 = property class="DigNum (严格)"(reference=w738) -> ("Value"=w737:u16)  [unwired: 1 in, 2 out]
        n436 = Not Equal?(x=w747, y=T13."待机") -> (x != y?=w746:bool)
        n437 = Greater Or Equal?(x=w737, y=u16 5) -> (x >= y?=w734:bool)
        n438 = Select(t="", s=w746, f="质控单元启动采样\n判断质控单元采样是否启动成功" ("State(s) In (\"\")")) -> (s? t:f=w743:string)
        n439 = Select(t="流程结束" ("State(s) In (\"\")"), s=w734, f=w743) -> (s? t:f=w741:string)
        n440 = case shown="真" w734 {
          tunnel: w733 -> [_ w752]
          frame False {
          }
          frame True {
            w751 = "质控单元采样启动失败" ("日志信息")
            n441 = call "启动日志.vi"("日志信息"=w751, "Slave ID"=w752) -> ()  [unwired: 9 in, 1 out]
            n442 = call "报警信息记录.vi"("报警信息"=w751, "Slave ID"=w752) -> ()  [unwired: 9 in, 1 out]
          }
        }
        n443 = call "Add State to Queue.vi"("State(s) In Front (\"\")"=w741, "State(s) In (\"\")"=w750) -> ("States Out"=w749:string)  [unwired: 13 in]
      }
      frame "判断质控单元加标是否启动成功" {
        n444 = case shown="\"CODCr\"" w765 {
          tunnel: [T13."异常停机" ("运行状态") w786 w788 w790 w792 w794] -> w779
          frame "null", Default {
          }
          frame "氨氮" {
            n445 = global read "ZK非断电保存全局变量.vi" "氨氮质控仪器状态"() -> (w787:T19)
            n446 = Unbundle By Name(w787) -> ("运行状态"=w786:T13)
          }
          frame "总磷" {
            n447 = global read "ZK非断电保存全局变量.vi" "总磷质控仪器状态"() -> (w789:T19)
            n448 = Unbundle By Name(w789) -> ("运行状态"=w788:T13)
          }
          frame "总氮" {
            n449 = global read "ZK非断电保存全局变量.vi" "总氮质控仪器状态"() -> (w791:T19)
            n450 = Unbundle By Name(w791) -> ("运行状态"=w790:T13)
          }
          frame "CODMn" {
            n451 = global read "ZK非断电保存全局变量.vi" "CODMn质控仪器状态"() -> (w793:T19)
            n452 = Unbundle By Name(w793) -> ("运行状态"=w792:T13)
          }
          frame "CODCr" {
            n453 = global read "ZK非断电保存全局变量.vi" "CODCr质控仪器状态"() -> (w795:T19)
            n454 = Unbundle By Name(w795) -> ("运行状态"=w794:T13)
          }
        }
        n455 = Index Array(array=w771, index=3 ("索引")) -> (element=w770:refnum<vi>)
        n456 = property class="DigNum (严格)"(reference=w770) -> ("Value"=w769:u16)  [unwired: 1 in, 2 out]
        n457 = call "启动日志.vi"("日志信息"=w767, "Slave ID"=w765) -> ()  [unwired: 9 in, 1 out]
        n458 = Greater Or Equal?(x=w769, y=u16 5) -> (x >= y?=w766:bool)
        n459 = Not Equal?(x=w779, y=T13."待机") -> (x != y?=w778:bool)
        n460 = Select(t="", s=w778, f="质控单元启动加标\n判断质控单元加标是否启动成功" ("State(s) In (\"\")")) -> (s? t:f=w775:string)
        n461 = Select(t="流程结束" ("State(s) In (\"\")"), s=w766, f=w775) -> (s? t:f=w773:string)
        n462 = case shown="真" w766 {
          tunnel: w765 -> [_ w784]
          frame False {
          }
          frame True {
            w783 = "质控单元加标启动失败" ("日志信息")
            n463 = call "启动日志.vi"("日志信息"=w783, "Slave ID"=w784) -> ()  [unwired: 9 in, 1 out]
            n464 = call "报警信息记录.vi"("报警信息"=w783, "Slave ID"=w784) -> ()  [unwired: 9 in, 1 out]
          }
        }
        n465 = call "Add State to Queue.vi"("State(s) In Front (\"\")"=w773, "State(s) In (\"\")"=w782) -> ("States Out"=w781:string)  [unwired: 13 in]
      }
      frame "判断质控单元排液是否启动成功" {
        n466 = Index Array(array=w803, index=4 ("索引")) -> (element=w802:refnum<vi>)
        n467 = case shown="\"CODCr\"" w797 {
          tunnel: [T13."异常停机" ("运行状态") w818 w820 w822 w824 w826] -> w811
          frame "null", Default {
          }
          frame "氨氮" {
            n468 = global read "ZK非断电保存全局变量.vi" "氨氮质控仪器状态"() -> (w819:T19)
            n469 = Unbundle By Name(w819) -> ("运行状态"=w818:T13)
          }
          frame "总磷" {
            n470 = global read "ZK非断电保存全局变量.vi" "总磷质控仪器状态"() -> (w821:T19)
            n471 = Unbundle By Name(w821) -> ("运行状态"=w820:T13)
          }
          frame "总氮" {
            n472 = global read "ZK非断电保存全局变量.vi" "总氮质控仪器状态"() -> (w823:T19)
            n473 = Unbundle By Name(w823) -> ("运行状态"=w822:T13)
          }
          frame "CODMn" {
            n474 = global read "ZK非断电保存全局变量.vi" "CODMn质控仪器状态"() -> (w825:T19)
            n475 = Unbundle By Name(w825) -> ("运行状态"=w824:T13)
          }
          frame "CODCr" {
            n476 = global read "ZK非断电保存全局变量.vi" "CODCr质控仪器状态"() -> (w827:T19)
            n477 = Unbundle By Name(w827) -> ("运行状态"=w826:T13)
          }
        }
        n478 = property class="DigNum (严格)"(reference=w802) -> ("Value"=w801:u16)  [unwired: 1 in, 2 out]
        n479 = call "启动日志.vi"("日志信息"=w799, "Slave ID"=w797) -> ()  [unwired: 9 in, 1 out]
        n480 = Greater Or Equal?(x=w801, y=u16 5) -> (x >= y?=w798:bool)
        n481 = Not Equal?(x=w811, y=T13."待机") -> (x != y?=w810:bool)
        n482 = Select(t="", s=w810, f="质控单元启动排液\n判断质控单元排液是否启动成功" ("State(s) In (\"\")")) -> (s? t:f=w807:string)
        n483 = Select(t="流程结束" ("State(s) In (\"\")"), s=w798, f=w807) -> (s? t:f=w805:string)
        n484 = case shown="真" w798 {
          tunnel: w797 -> [_ w816]
          frame False {
          }
          frame True {
            w815 = "质控单元排液启动失败" ("日志信息")
            n485 = call "启动日志.vi"("日志信息"=w815, "Slave ID"=w816) -> ()  [unwired: 9 in, 1 out]
            n486 = call "报警信息记录.vi"("报警信息"=w815, "Slave ID"=w816) -> ()  [unwired: 9 in, 1 out]
          }
        }
        n487 = call "Add State to Queue.vi"("State(s) In Front (\"\")"=w805, "State(s) In (\"\")"=w814) -> ("States Out"=w813:string)  [unwired: 13 in]
      }
      frame "质控单元采样中", "质控单元加标中", "质控单元润洗中" {
        n488 = case shown="\"CODCr\"" w830 {
          tunnel: [T13."待机" ("运行状态") w851 w853 w855 w857 w859] -> w835
          frame "null", Default {
          }
          frame "氨氮" {
            n489 = global read "ZK非断电保存全局变量.vi" "氨氮质控仪器状态"() -> (w852:T19)
            n490 = Unbundle By Name(w852) -> ("运行状态"=w851:T13)
          }
          frame "总磷" {
            n491 = global read "ZK非断电保存全局变量.vi" "总磷质控仪器状态"() -> (w854:T19)
            n492 = Unbundle By Name(w854) -> ("运行状态"=w853:T13)
          }
          frame "总氮" {
            n493 = global read "ZK非断电保存全局变量.vi" "总氮质控仪器状态"() -> (w856:T19)
            n494 = Unbundle By Name(w856) -> ("运行状态"=w855:T13)
          }
          frame "CODMn" {
            n495 = global read "ZK非断电保存全局变量.vi" "CODMn质控仪器状态"() -> (w858:T19)
            n496 = Unbundle By Name(w858) -> ("运行状态"=w857:T13)
          }
          frame "CODCr" {
            n497 = global read "ZK非断电保存全局变量.vi" "CODCr质控仪器状态"() -> (w860:T19)
            n498 = Unbundle By Name(w860) -> ("运行状态"=w859:T13)
          }
        }
        n499 = case shown="真" w828 {
          tunnel: w830 -> [_ w849]
          tunnel: w836 -> [_ w848]
          frame False {
          }
          frame True {
            n500 = call "启动日志.vi"("日志信息"=w848, "Slave ID"=w849) -> ()  [unwired: 9 in, 1 out]
          }
        }
        n501 = Equal?(x=w835, y=T13."等待取样") -> (x = y?=w841:bool)
        n502 = Select(t="", s=w841, f=w836) -> (s? t:f=w839:string)
        n503 = Equal?(x=w835, y=T13."待机") -> (x = y?=w833:bool)
        n504 = Equal?(x=w835, y=T13."异常停机") -> (x = y?=w832:bool)
        n505 = Or(x=w832, y=w833) -> (x .or. y?=w831:bool)
        n506 = Select(t="流程结束" ("State(s) In (\"\")"), s=w831, f=w839) -> (s? t:f=w837:string)
        n507 = case shown="真" w831 {
          tunnel: w830 -> [_ w847]
          frame False {
          }
          frame True {
            w846 = "质控单元流程中断" ("日志信息")
            n508 = call "启动日志.vi"("日志信息"=w846, "Slave ID"=w847) -> ()  [unwired: 9 in, 1 out]
            n509 = call "报警信息记录.vi"("报警信息"=w846, "Slave ID"=w847) -> ()  [unwired: 9 in, 1 out]
          }
        }
        n510 = call "Add State to Queue.vi"("State(s) In Front (\"\")"=w837, "State(s) In (\"\")"=w845) -> ("States Out"=w844:string)  [unwired: 13 in]
      }
      frame "质控单元排液中" {
        n511 = case shown="\"CODCr\"" w863 {
          tunnel: [T13."异常停机" ("运行状态") w881 w883 w885 w887 w889] -> w872
          frame "null", Default {
          }
          frame "氨氮" {
            n512 = global read "ZK非断电保存全局变量.vi" "氨氮质控仪器状态"() -> (w882:T19)
            n513 = Unbundle By Name(w882) -> ("运行状态"=w881:T13)
          }
          frame "总磷" {
            n514 = global read "ZK非断电保存全局变量.vi" "总磷质控仪器状态"() -> (w884:T19)
            n515 = Unbundle By Name(w884) -> ("运行状态"=w883:T13)
          }
          frame "总氮" {
            n516 = global read "ZK非断电保存全局变量.vi" "总氮质控仪器状态"() -> (w886:T19)
            n517 = Unbundle By Name(w886) -> ("运行状态"=w885:T13)
          }
          frame "CODMn" {
            n518 = global read "ZK非断电保存全局变量.vi" "CODMn质控仪器状态"() -> (w888:T19)
            n519 = Unbundle By Name(w888) -> ("运行状态"=w887:T13)
          }
          frame "CODCr" {
            n520 = global read "ZK非断电保存全局变量.vi" "CODCr质控仪器状态"() -> (w890:T19)
            n521 = Unbundle By Name(w890) -> ("运行状态"=w889:T13)
          }
        }
        n522 = case shown="真" w861 {
          tunnel: w863 -> [_ w879]
          tunnel: w865 -> [_ w878]
          frame False {
          }
          frame True {
            n523 = call "启动日志.vi"("日志信息"=w878, "Slave ID"=w879) -> ()  [unwired: 9 in, 1 out]
          }
        }
        n524 = Equal?(x=w872, y=T13."待机") -> (x = y?=w870:bool)
        n525 = Select(t="", s=w870, f=w865) -> (s? t:f=w868:string)
        n526 = Equal?(x=w872, y=T13."异常停机") -> (x = y?=w864:bool)
        n527 = Select(t="流程结束" ("State(s) In (\"\")"), s=w864, f=w868) -> (s? t:f=w866:string)
        n528 = case shown="真" w864 {
          tunnel: w863 -> [_ w877]
          frame False {
          }
          frame True {
            w876 = "质控单元排液流程中断" ("日志信息")
            n529 = call "启动日志.vi"("日志信息"=w876, "Slave ID"=w877) -> ()  [unwired: 9 in, 1 out]
            n530 = call "报警信息记录.vi"("报警信息"=w876, "Slave ID"=w877) -> ()  [unwired: 9 in, 1 out]
          }
        }
        n531 = call "Add State to Queue.vi"("State(s) In Front (\"\")"=w866, "State(s) In (\"\")"=w875) -> ("States Out"=w874:string)  [unwired: 13 in]
      }
      frame "质控单元搅拌中" {
        n532 = case shown="真" w891 {
          tunnel: w892 -> [_ w905]
          tunnel: w897 -> [_ w904]
          frame False {
          }
          frame True {
            n533 = call "启动日志.vi"("日志信息"=w904, "Slave ID"=w905) -> ()  [unwired: 9 in, 1 out]
          }
        }
        n534 = Greater Or Equal?(x=w895, y=15) -> (x >= y?=w893:bool)
        n535 = case shown="真" w893 {
          tunnel: w892 -> [_ w901]
          frame False {
          }
          frame True {
            n536 = call "ZK组合命令区.vi"("是否启用通讯通知"=FALSE, "组合命令区"=质控组合命令区."停止", "Slave ID"=w901) -> ()  [unwired: 8 in, 1 out]
          }
        }
        n537 = Select(t="", s=w893, f=w897) -> (s? t:f=w896:string)
        n538 = call "Add State to Queue.vi"("State(s) In Front (\"\")"=w896, "State(s) In (\"\")"=w900) -> ("States Out"=w899:string)  [unwired: 13 in]
      }
      frame "-------------------# 仪器测试流程 #-------------------" {
        n539 = call "Add State to Queue.vi"("State(s) In (\"\")"=w908) -> ("States Out"=w907:string)  [unwired: 14 in]
      }
      frame "启动仪器水样测试" {
        n540 = case shown="\"总氮\"" w913 {
          tunnel: enum16{"水样测试", "平行样测试", "加标回收", "停止"}."水样测试" ("控制命令") -> [_ w922 w923 w924 w925 w926]
          frame "null", Default {
          }
          frame "氨氮" {
            n541 = call "氨氮启动器.vi"("控制命令"=w922) -> ()  [unwired: 11 in]
          }
          frame "总磷" {
            n542 = call "总磷启动器.vi"("控制命令"=w923) -> ()  [unwired: 11 in]
          }
          frame "总氮" {
            n543 = call "总氮启动器.vi"("控制命令"=w924) -> ()  [unwired: 11 in]
          }
          frame "CODMn" {
            n544 = call "CODmn启动器.vi"("控制命令"=w925) -> ()  [unwired: 11 in]
          }
          frame "CODCr" {
            n545 = call "CODcr启动器.vi"("控制命令"=w926) -> ()  [unwired: 11 in]
          }
        }
        n546 = Index Array(array=w916, index=5 ("索引")) -> (element=w915:refnum<vi>)
        n547 = property class="DigNum (严格)"(reference=w915) -> (reference out=w919:refnum<vi>, "Value"=w918:u16)  [unwired: 1 in, 1 out]
        n548 = Get Date/Time In Seconds() -> (seconds since 1Jan1904=→"水样测试启动时间":timestamp)
        n549 = call "启动日志.vi"("日志信息"=w912, "Slave ID"=w913) -> ()  [unwired: 9 in, 1 out]
        n550 = Increment(x=w918) -> (x+1=w917:u16)
        n551 = property class="DigNum (严格)"(reference=w919, "Value"=w917) -> ()  [unwired: 1 in, 2 out]
        n552 = call "Add State to Queue.vi"("State(s) In (\"\")"=w921) -> ("States Out"=w920:string)  [unwired: 14 in]
      }
      frame "等待仪器空闲" {
        n553 = case shown="\"总磷\"" w930 {
          tunnel: w929 -> [_ w935]
          tunnel: [_ w934] -> w928
          frame "null", Default {
          }
          frame "总磷" {
            n554 = global read "系统交互.vi" "总磷总氮类型"() -> (w936:enum16{"单模块", "二合一模块"})
            n555 = case shown="\"二合一模块\"" w936 {
              tunnel: w935 -> [_ w939]
              tunnel: [_ w938] -> w934
              frame "单模块", Default {
              }
              frame "二合一模块" {
                n556 = global read "ZK非断电保存全局变量.vi" "流程运行状态标记位"() -> (w941:T7)
                n557 = Unbundle By Name(w941) -> ("总氮"=w940:bool)
                n558 = Select(t=w939, s=w940, f="") -> (s? t:f=w938:string)
              }
            }
          }
        }
        n559 = case shown="真" w927 {
          tunnel: w930 -> [_ w943]
          tunnel: w929 -> [_ w942]
          frame False {
          }
          frame True {
            n560 = call "启动日志.vi"("日志信息"=w942, "Slave ID"=w943) -> ()  [unwired: 9 in, 1 out]
          }
        }
        n561 = call "Add State to Queue.vi"("State(s) In Front (\"\")"=w928, "State(s) In (\"\")"=w933) -> ("States Out"=w932:string)  [unwired: 13 in]
      }
      frame "启动仪器加标回收测试" {
        n562 = case shown="\"CODMn\"" w948 {
          tunnel: enum16{"水样测试", "平行样测试", "加标回收", "停止"}."加标回收" ("控制命令") -> [_ w957 w958 w959 w960 w961]
          frame "null", Default {
          }
          frame "氨氮" {
            n563 = call "氨氮启动器.vi"("控制命令"=w957) -> ()  [unwired: 11 in]
          }
          frame "总磷" {
            n564 = call "总磷启动器.vi"("控制命令"=w958) -> ()  [unwired: 11 in]
          }
          frame "总氮" {
            n565 = call "总氮启动器.vi"("控制命令"=w959) -> ()  [unwired: 11 in]
          }
          frame "CODMn" {
            n566 = call "CODmn启动器.vi"("控制命令"=w960) -> ()  [unwired: 11 in]
          }
          frame "CODCr" {
            n567 = call "CODcr启动器.vi"("控制命令"=w961) -> ()  [unwired: 11 in]
          }
        }
        n568 = Index Array(array=w951, index=6 ("索引")) -> (element=w950:refnum<vi>)
        n569 = property class="DigNum (严格)"(reference=w950) -> (reference out=w954:refnum<vi>, "Value"=w953:u16)  [unwired: 1 in, 1 out]
        n570 = call "启动日志.vi"("日志信息"=w947, "Slave ID"=w948) -> ()  [unwired: 9 in, 1 out]
        n571 = Get Date/Time In Seconds() -> (seconds since 1Jan1904=→"加标回收启动时间":timestamp)
        n572 = Increment(x=w953) -> (x+1=w952:u16)
        n573 = property class="DigNum (严格)"(reference=w954, "Value"=w952) -> ()  [unwired: 1 in, 2 out]
        n574 = call "Add State to Queue.vi"("State(s) In (\"\")"=w956) -> ("States Out"=w955:string)  [unwired: 14 in]
      }
      frame "启动仪器平行样测试" {
        n575 = case shown="\"总磷\"" w966 {
          tunnel: enum16{"水样测试", "平行样测试", "加标回收", "停止"}."平行样测试" ("控制命令") -> [_ w975 w976 w977 w978 w979]
          frame "null", Default {
          }
          frame "氨氮" {
            n576 = call "氨氮启动器.vi"("控制命令"=w975) -> ()  [unwired: 11 in]
          }
          frame "总磷" {
            n577 = call "总磷启动器.vi"("控制命令"=w976) -> ()  [unwired: 11 in]
          }
          frame "总氮" {
            n578 = call "总氮启动器.vi"("控制命令"=w977) -> ()  [unwired: 11 in]
          }
          frame "CODMn" {
            n579 = call "CODmn启动器.vi"("控制命令"=w978) -> ()  [unwired: 11 in]
          }
          frame "CODCr" {
            n580 = call "CODcr启动器.vi"("控制命令"=w979) -> ()  [unwired: 11 in]
          }
        }
        n581 = Index Array(array=w969, index=6 ("索引")) -> (element=w968:refnum<vi>)
        n582 = property class="DigNum (严格)"(reference=w968) -> (reference out=w972:refnum<vi>, "Value"=w971:u16)  [unwired: 1 in, 1 out]
        n583 = call "启动日志.vi"("日志信息"=w965, "Slave ID"=w966) -> ()  [unwired: 9 in, 1 out]
        n584 = Get Date/Time In Seconds() -> (seconds since 1Jan1904=→"平行样启动时间":timestamp)
        n585 = Increment(x=w971) -> (x+1=w970:u16)
        n586 = property class="DigNum (严格)"(reference=w972, "Value"=w970) -> ()  [unwired: 1 in, 2 out]
        n587 = call "Add State to Queue.vi"("State(s) In (\"\")"=w974) -> ("States Out"=w973:string)  [unwired: 14 in]
      }
      frame "exit" {
        n588 = flat-sequence {
          tunnel: w982 -> [w987]
          frame #0 {
            n589 = global read "ZK非断电保存全局变量.vi" "流程运行状态标记位"() -> (w988:T7)
            n590 = case shown="\"氨氮\"" w987 {
              tunnel: w988 -> [_ w991 w992 w995 w998 w1001]
              frame "null", Default {
              }
              frame "氨氮" {
                n591 = Bundle By Name(cluster=w991, "氨氮"=FALSE) -> (w990:T7)
                n592 = global write "ZK非断电保存全局变量.vi" "流程运行状态标记位"(w990) -> ()
              }
              frame "总磷" {
                n593 = Bundle By Name(cluster=w992, "总磷"=FALSE ("氨氮")) -> (w994:T7)
                n594 = global write "ZK非断电保存全局变量.vi" "流程运行状态标记位"(w994) -> ()
              }
              frame "总氮" {
                n595 = Bundle By Name(cluster=w995, "总氮"=FALSE ("氨氮")) -> (w997:T7)
                n596 = global write "ZK非断电保存全局变量.vi" "流程运行状态标记位"(w997) -> ()
              }
              frame "CODMn" {
                n597 = Bundle By Name(cluster=w998, "CODMn"=FALSE ("氨氮")) -> (w1000:T7)
                n598 = global write "ZK非断电保存全局变量.vi" "流程运行状态标记位"(w1000) -> ()
              }
              frame "CODCr" {
                n599 = Bundle By Name(cluster=w1001, "CODCr"=FALSE ("氨氮")) -> (w1003:T7)
                n600 = global write "ZK非断电保存全局变量.vi" "流程运行状态标记位"(w1003) -> ()
              }
            }
          }
          frame #1 {
            n601 = global read "ZK非断电保存全局变量.vi" "流程运行状态标记位"() -> (w1007:T7)
            n602 = Cluster To Array(cluster=w1007) -> (array=w1006:bool[])
            n603 = Boolean Array To Number(Boolean array=w1006) -> (number=w1005:u32)
            n604 = Equal To 0?(x=w1005) -> (x = 0?=w1004:bool)
            n605 = case shown="真" w1004 {
              frame False {
              }
              frame True {
                n606 = call "采配水启动器.vi"("启动/停止命令"=T9."停止") -> ()  [unwired: 10 in, 1 out]
              }
            }
          }
        }
        n607 = case shown="\"CODMn\"" w982 {
          tunnel: enum16{"水样测试", "平行样测试", "加标回收", "停止"}."停止" ("控制命令") -> [_ w1009 w1010 w1011 w1012 w1013]
          frame "null", Default {
          }
          frame "氨氮" {
            n608 = call "氨氮启动器.vi"("控制命令"=w1009) -> ()  [unwired: 11 in]
          }
          frame "总磷" {
            n609 = call "总磷启动器.vi"("控制命令"=w1010) -> ()  [unwired: 11 in]
          }
          frame "总氮" {
            n610 = call "总氮启动器.vi"("控制命令"=w1011) -> ()  [unwired: 11 in]
          }
          frame "CODMn" {
            n611 = call "CODmn启动器.vi"("控制命令"=w1012) -> ()  [unwired: 11 in]
          }
          frame "CODCr" {
            n612 = call "CODcr启动器.vi"("控制命令"=w1013) -> ()  [unwired: 11 in]
          }
        }
        n613 = call "启动日志.vi"("日志信息"=w984, "Slave ID"=w982) -> ()  [unwired: 9 in, 1 out]
        n614 = call "Add State to Queue.vi"("State(s) In Front (\"\")"="流程结束" ("State(s) In Front (\"\")"), "State(s) In (\"\")"=w986) -> ("States Out"=w985:string)  [unwired: 13 in]
      }
      frame "判断仪器水样是否启动成功" {
        n615 = case shown="\"CODCr\"" w1015 {
          tunnel: [T14."空闲" ("工作状态") w1037 w1039 w1041 w1043 w1045] -> w1030
          frame "null", Default {
          }
          frame "氨氮" {
            w1036 = u16 3 items=["总磷"=1, "总氮"=2, "氨氮"=3, "CODMn"=21] ("站号")
            n616 = call "获取仪器仪表状态.vi"("站号"=w1036) -> ("工作状态"=w1037:T14)  [unwired: 10 in]
          }
          frame "总磷" {
            w1038 = u16 1 items=["总磷"=1, "总氮"=2, "氨氮"=3, "CODMn"=21] ("站号")
            n617 = call "获取仪器仪表状态.vi"("站号"=w1038) -> ("工作状态"=w1039:T14)  [unwired: 10 in]
          }
          frame "总氮" {
            w1040 = u16 2 items=["总磷"=1, "总氮"=2, "氨氮"=3, "CODMn"=21] ("站号")
            n618 = call "获取仪器仪表状态.vi"("站号"=w1040) -> ("工作状态"=w1041:T14)  [unwired: 10 in]
          }
          frame "CODMn" {
            w1042 = u16 21 items=["总磷"=1, "总氮"=2, "氨氮"=3, "CODMn"=21] ("站号")
            n619 = call "获取仪器仪表状态.vi"("站号"=w1042) -> ("工作状态"=w1043:T14)  [unwired: 10 in]
          }
          frame "CODCr" {
            w1044 = u16 22 items=["总磷"=1, "总氮"=2, "氨氮"=3, "CODMn"=21, "CODcr"=22] ("站号")
            n620 = call "获取仪器仪表状态.vi"("站号"=w1044) -> ("工作状态"=w1045:T14)  [unwired: 10 in]
          }
        }
        n621 = Index Array(array=w1021, index=5 ("索引")) -> (element=w1020:refnum<vi>)
        n622 = call "启动日志.vi"("日志信息"=w1017, "Slave ID"=w1015) -> ()  [unwired: 9 in, 1 out]
        n623 = property class="DigNum (严格)"(reference=w1020) -> ("Value"=w1019:u16)  [unwired: 1 in, 2 out]
        n624 = Greater Or Equal?(x=w1019, y=u16 5) -> (x >= y?=w1016:bool)
        n625 = Equal?(x=w1030, y=T14."空闲") -> (x = y?=w1028:bool)
        n626 = Select(t="启动仪器水样测试\n判断仪器水样是否启动成功" ("State(s) In (\"\")"), s=w1028, f="") -> (s? t:f=w1023:string)
        n627 = case shown="真" w1016 {
          tunnel: w1015 -> [_ w1034]
          frame False {
          }
          frame True {
            w1033 = "水样测试启动失败" ("日志信息")
            n628 = call "启动日志.vi"("日志信息"=w1033, "Slave ID"=w1034) -> ()  [unwired: 9 in, 1 out]
            n629 = call "报警信息记录.vi"("报警信息"=w1033, "Slave ID"=w1034) -> ()  [unwired: 9 in, 1 out]
          }
        }
        n630 = Select(t="流程结束" ("State(s) In (\"\")"), s=w1016, f=w1023) -> (s? t:f=w1022:string)
        n631 = call "Add State to Queue.vi"("State(s) In Front (\"\")"=w1022, "State(s) In (\"\")"=w1032) -> ("States Out"=w1031:string)  [unwired: 13 in]
      }
      frame "判断仪器加标是否启动成功" {
        n632 = case shown="\"CODCr\"" w1047 {
          tunnel: [T14."空闲" ("工作状态") w1069 w1071 w1073 w1075 w1077] -> w1050
          frame "null", Default {
          }
          frame "氨氮" {
            w1068 = u16 3 items=["总磷"=1, "总氮"=2, "氨氮"=3, "CODMn"=21] ("站号")
            n633 = call "获取仪器仪表状态.vi"("站号"=w1068) -> ("工作状态"=w1069:T14)  [unwired: 10 in]
          }
          frame "总磷" {
            w1070 = u16 1 items=["总磷"=1, "总氮"=2, "氨氮"=3, "CODMn"=21] ("站号")
            n634 = call "获取仪器仪表状态.vi"("站号"=w1070) -> ("工作状态"=w1071:T14)  [unwired: 10 in]
          }
          frame "总氮" {
            w1072 = u16 2 items=["总磷"=1, "总氮"=2, "氨氮"=3, "CODMn"=21] ("站号")
            n635 = call "获取仪器仪表状态.vi"("站号"=w1072) -> ("工作状态"=w1073:T14)  [unwired: 10 in]
          }
          frame "CODMn" {
            w1074 = u16 21 items=["总磷"=1, "总氮"=2, "氨氮"=3, "CODMn"=21] ("站号")
            n636 = call "获取仪器仪表状态.vi"("站号"=w1074) -> ("工作状态"=w1075:T14)  [unwired: 10 in]
          }
          frame "CODCr" {
            w1076 = u16 22 items=["总磷"=1, "总氮"=2, "氨氮"=3, "CODMn"=21, "CODcr"=22] ("站号")
            n637 = call "获取仪器仪表状态.vi"("站号"=w1076) -> ("工作状态"=w1077:T14)  [unwired: 10 in]
          }
        }
        n638 = Index Array(array=w1054, index=6 ("索引")) -> (element=w1053:refnum<vi>)
        n639 = call "启动日志.vi"("日志信息"=w1049, "Slave ID"=w1047) -> ()  [unwired: 9 in, 1 out]
        n640 = property class="DigNum (严格)"(reference=w1053) -> ("Value"=w1052:u16)  [unwired: 1 in, 2 out]
        n641 = Greater Or Equal?(x=w1052, y=u16 5) -> (x >= y?=w1048:bool)
        n642 = Equal?(x=w1050, y=T14."空闲") -> (x = y?=w1061:bool)
        n643 = Select(t="启动仪器加标回收测试\n判断仪器加标是否启动成功" ("State(s) In (\"\")"), s=w1061, f="") -> (s? t:f=w1056:string)
        n644 = case shown="真" w1048 {
          tunnel: w1047 -> [_ w1066]
          frame False {
          }
          frame True {
            w1065 = "加标回收启动失败" ("日志信息")
            n645 = call "启动日志.vi"("日志信息"=w1065, "Slave ID"=w1066) -> ()  [unwired: 9 in, 1 out]
            n646 = call "报警信息记录.vi"("报警信息"=w1065, "Slave ID"=w1066) -> ()  [unwired: 9 in, 1 out]
          }
        }
        n647 = Select(t="流程结束" ("State(s) In (\"\")"), s=w1048, f=w1056) -> (s? t:f=w1055:string)
        n648 = call "Add State to Queue.vi"("State(s) In Front (\"\")"=w1055, "State(s) In (\"\")"=w1064) -> ("States Out"=w1063:string)  [unwired: 13 in]
      }
      frame "判断仪器平行样是否启动成功" {
        n649 = case shown="\"CODCr\"" w1079 {
          tunnel: [T14."空闲" ("工作状态") w1101 w1103 w1105 w1107 w1109] -> w1082
          frame "null", Default {
          }
          frame "氨氮" {
            w1100 = u16 3 items=["总磷"=1, "总氮"=2, "氨氮"=3, "CODMn"=21] ("站号")
            n650 = call "获取仪器仪表状态.vi"("站号"=w1100) -> ("工作状态"=w1101:T14)  [unwired: 10 in]
          }
          frame "总磷" {
            w1102 = u16 1 items=["总磷"=1, "总氮"=2, "氨氮"=3, "CODMn"=21] ("站号")
            n651 = call "获取仪器仪表状态.vi"("站号"=w1102) -> ("工作状态"=w1103:T14)  [unwired: 10 in]
          }
          frame "总氮" {
            w1104 = u16 2 items=["总磷"=1, "总氮"=2, "氨氮"=3, "CODMn"=21] ("站号")
            n652 = call "获取仪器仪表状态.vi"("站号"=w1104) -> ("工作状态"=w1105:T14)  [unwired: 10 in]
          }
          frame "CODMn" {
            w1106 = u16 21 items=["总磷"=1, "总氮"=2, "氨氮"=3, "CODMn"=21] ("站号")
            n653 = call "获取仪器仪表状态.vi"("站号"=w1106) -> ("工作状态"=w1107:T14)  [unwired: 10 in]
          }
          frame "CODCr" {
            w1108 = u16 22 items=["总磷"=1, "总氮"=2, "氨氮"=3, "CODMn"=21, "CODcr"=22] ("站号")
            n654 = call "获取仪器仪表状态.vi"("站号"=w1108) -> ("工作状态"=w1109:T14)  [unwired: 10 in]
          }
        }
        n655 = Index Array(array=w1086, index=6 ("索引")) -> (element=w1085:refnum<vi>)
        n656 = call "启动日志.vi"("日志信息"=w1081, "Slave ID"=w1079) -> ()  [unwired: 9 in, 1 out]
        n657 = property class="DigNum (严格)"(reference=w1085) -> ("Value"=w1084:u16)  [unwired: 1 in, 2 out]
        n658 = Greater Or Equal?(x=w1084, y=u16 5) -> (x >= y?=w1080:bool)
        n659 = Equal?(x=w1082, y=T14."空闲") -> (x = y?=w1093:bool)
        n660 = Select(t="启动仪器平行样测试\n判断仪器平行样是否启动成功" ("State(s) In (\"\")"), s=w1093, f="") -> (s? t:f=w1088:string)
        n661 = case shown="真" w1080 {
          tunnel: w1079 -> [_ w1098]
          frame False {
          }
          frame True {
            w1097 = "平行样启动失败" ("日志信息")
            n662 = call "启动日志.vi"("日志信息"=w1097, "Slave ID"=w1098) -> ()  [unwired: 9 in, 1 out]
            n663 = call "报警信息记录.vi"("报警信息"=w1097, "Slave ID"=w1098) -> ()  [unwired: 9 in, 1 out]
          }
        }
        n664 = Select(t="流程结束" ("State(s) In (\"\")"), s=w1080, f=w1088) -> (s? t:f=w1087:string)
        n665 = call "Add State to Queue.vi"("State(s) In Front (\"\")"=w1087, "State(s) In (\"\")"=w1096) -> ("States Out"=w1095:string)  [unwired: 13 in]
      }
      frame "仪器加标回收测试中", "仪器平行样测试中", "仪器水样测试中" {
        n666 = case shown="\"CODCr\"" w1113 {
          tunnel: [T14."空闲" ("工作状态") w1123 w1125 w1127 w1129 w1131] -> w1112
          frame "null", Default {
          }
          frame "氨氮" {
            w1122 = u16 3 items=["总磷"=1, "总氮"=2, "氨氮"=3, "CODMn"=21] ("站号")
            n667 = call "获取仪器仪表状态.vi"("站号"=w1122) -> ("工作状态"=w1123:T14)  [unwired: 10 in]
          }
          frame "总磷" {
            w1124 = u16 1 items=["总磷"=1, "总氮"=2, "氨氮"=3, "CODMn"=21] ("站号")
            n668 = call "获取仪器仪表状态.vi"("站号"=w1124) -> ("工作状态"=w1125:T14)  [unwired: 10 in]
          }
          frame "总氮" {
            w1126 = u16 2 items=["总磷"=1, "总氮"=2, "氨氮"=3, "CODMn"=21] ("站号")
            n669 = call "获取仪器仪表状态.vi"("站号"=w1126) -> ("工作状态"=w1127:T14)  [unwired: 10 in]
          }
          frame "CODMn" {
            w1128 = u16 21 items=["总磷"=1, "总氮"=2, "氨氮"=3, "CODMn"=21] ("站号")
            n670 = call "获取仪器仪表状态.vi"("站号"=w1128) -> ("工作状态"=w1129:T14)  [unwired: 10 in]
          }
          frame "CODCr" {
            w1130 = u16 22 items=["总磷"=1, "总氮"=2, "氨氮"=3, "CODMn"=21, "CODcr"=22] ("站号")
            n671 = call "获取仪器仪表状态.vi"("站号"=w1130) -> ("工作状态"=w1131:T14)  [unwired: 10 in]
          }
        }
        n672 = case shown="真" w1110 {
          tunnel: w1113 -> [_ w1133]
          tunnel: w1114 -> [_ w1132]
          frame False {
          }
          frame True {
            n673 = call "启动日志.vi"("日志信息"=w1132, "Slave ID"=w1133) -> ()  [unwired: 9 in, 1 out]
          }
        }
        n674 = Equal?(x=w1112, y=T14."空闲") -> (x = y?=w1117:bool)
        n675 = Select(t="", s=w1117, f=w1114) -> (s? t:f=w1115:string)
        n676 = call "Add State to Queue.vi"("State(s) In Front (\"\")"=w1115, "State(s) In (\"\")"=w1120) -> ("States Out"=w1119:string)  [unwired: 13 in]
      }
    }
  }
